vi "Coerce Value.vi"(8 "error in (no error)":errorcluster, 9 "Value":variant, 10 "ParamTags":T1, 11 "Rigol DG822 Pulse in":refnum<class "Rigol DG822 Pulse.lvclass">) -> (0 "error out":errorcluster, 1 "Coerced Value":variant, 3 "Rigol DG822 Pulse out":refnum<class "Rigol DG822 Pulse.lvclass">)   [LabVIEW 2021, in "Rigol DG822 UI.lvlib" / "Rigol DG822 Pulse.lvlib" / "Rigol DG822 Pulse.lvclass"]
uses:
  Rigol DG822 Pulse.lvclass
  Rigol DG822 UI/lib/controls.llb/WaveformParamTags.ctl
  Rigol DG822 UI/lib/controls.llb/FreqUnit.ctl
  Rigol DG822 UI/lib/controls.llb/PeriodUnit.ctl
  Rigol DG822 Pulse.lvclass/Rigol DG822 Pulse.ctl
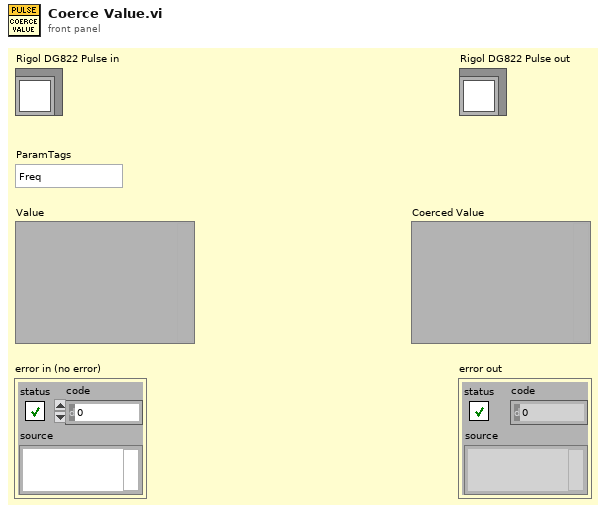
[diagram p1: front panel]
types:
  T1 = typedef "WaveformParamTags.ctl" = enum16{"Freq", "Period", "Ampl", "HighL", "Offset", "LowL", "Phase", "Duty", "Width", "RisEdge", "FallEdge"}
  T2 = typedef "FreqUnit.ctl" = enum32{"No Selection", "MHz", "kHz", "Hz", "mHz", "uHz"}
  T3 = cluster{"Freq":dbl, "FreqUnit":T2, "FreqUnitPrecision":dbl}
  T4 = typedef "PeriodUnit.ctl" = enum32{"No Selection", "s", "ms", "us", "ns"}
  T5 = cluster{"Period":dbl, "PeriodUnit":T4, "PeriodUnitPrecision":dbl}
  T6 = cluster{"Ampl":dbl, "AmplUnit":enum32{"No Selection", "Vpp", "mVpp"}, "AmplUnitPrecision":dbl}
  T7 = cluster{"HighL":dbl, "HighLUnit":enum32{"No Selection", "V", "mV"}, "HighLUnitPrecision":dbl}
  T8 = cluster{"Offset":dbl, "OffsetUnit":enum32{"No Selection", "Vdc", "mVdc"}, "OffsetUnitPrecision":dbl}
  T9 = cluster{"LowL":dbl, "LowLUnit":enum32{"No Selection", "V", "mV"}, "LowLUnitPrecision":dbl}
  T10 = cluster{"Phase":dbl, "PhaseUnit":enum32{"°"}, "PhaseUnitPrecision":dbl}
  T11 = cluster{"Duty":dbl, "DutyUnit":enum32{"%"}, "DutyUnitPrcs":dbl}
  T12 = cluster{"Width":dbl, "WidthUnit":enum32{"No Selection", "s", "ms", "us", "ns"}, "WidthUnitPrcs":dbl}
  T13 = cluster{"RisEdge":dbl, "RisEdgeUnit":enum32{"No Selection", "s", "ms", "us", "ns"}, "RisEdgeUnitPrcs":dbl}
  T14 = cluster{"FallEdge":dbl, "FallEdgeUnit":enum32{"No Selection", "s", "ms", "us", "ns"}, "FallEdgeUnitPrcs":dbl}
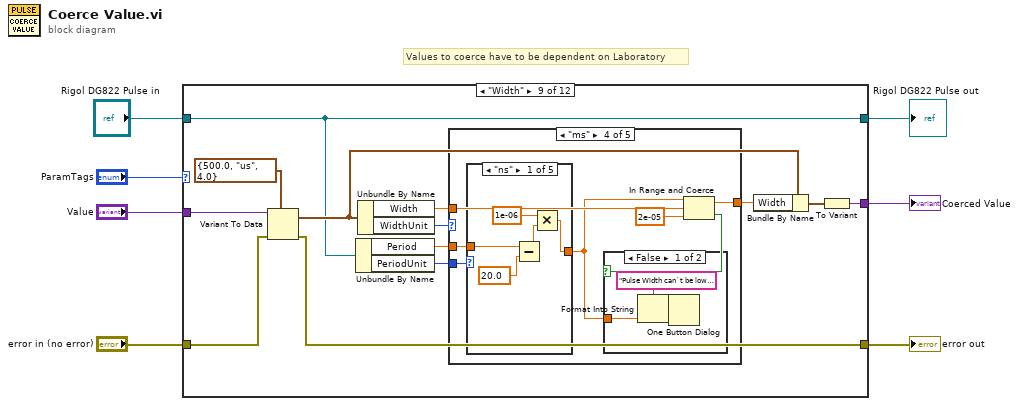
[diagram p0: block diagram]
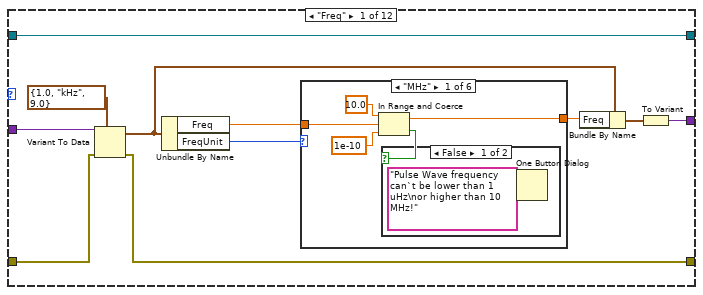
[diagram p2: hidden frame]
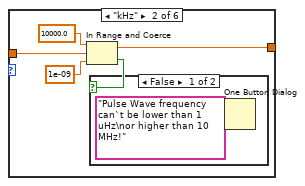
[diagram p4: hidden frame]
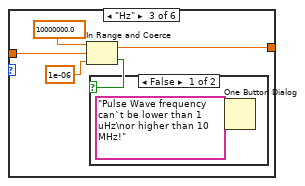
[diagram p6: hidden frame]
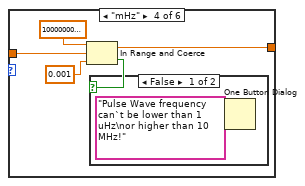
[diagram p8: hidden frame]
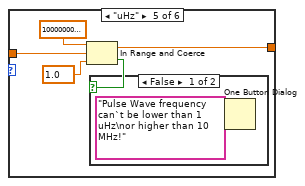
[diagram p10: hidden frame]
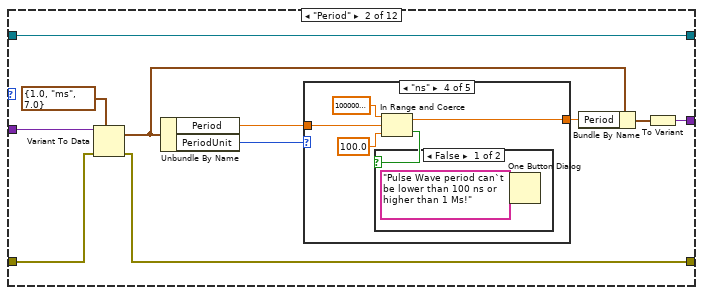
[diagram p13: hidden frame]
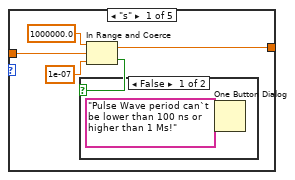
[diagram p14: hidden frame]
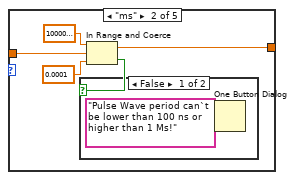
[diagram p16: hidden frame]
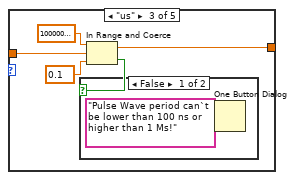
[diagram p18: hidden frame]
diagram:
  # "Values to coerce have to be dependent on Laboratory"
  n1 = case shown="\"Width\"" "ParamTags" {
    tunnel: "Value" -> [w14 w57 w93 w119 w167 w233 w279 w298 w370 w509 w1204 w1886]
    tunnel: "error in (no error)" -> [w12 w53 w90 w117 w165 w231 w276 w296 w368 w507 w1202 w1885]
    tunnel: [w11 w52 w89 w116 w164 w230 w275 w295 w367 w506 w1201 w1885] -> w4
    tunnel: [w9 w50 w87 w114 w162 w228 w273 w293 w365 w504 w1199 w1886] -> w1
    tunnel: "Rigol DG822 Pulse in" -> [w8 w54 w91 w112 w160 w227 w277 w291 w361 w502 w1198 w1887]
    tunnel: [w8 w54 w91 w112 w160 w227 w277 w291 w361 w502 w1198 w1887] -> w2
    frame "Freq" {
      n2 = Variant To Data(error in=w12, type=T3 {"Freq"=1.0, "FreqUnit"=enum."kHz", "FreqUnitPrecision"=9.0} ("Freq"), Variant=w14) -> (data=w13:T3, error out=w11:errorcluster)
      n3 = Unbundle By Name(w13) -> ("Freq"=w17:dbl, "FreqUnit"=w18:T2)
      n4 = case shown="\"MHz\"" w18 {
        tunnel: [w20 w26 w32 w38 w44 w49] -> w16
        tunnel: w17 -> [w21 w27 w33 w39 w45 w49]
        frame "MHz" {
          n5 = In Range and Coerce(upper limit=10.0, x=w21, lower limit=1e-10 ("t")) -> (coerced(x)=w20:dbl, In Range?=w19:bool)
          n6 = case shown="False" w19 {
            frame False {
              n7 = One Button Dialog(message="Pulse Wave frequency can`t be lower than 1 uHz\nor higher than 10 MHz!") -> ()  [unwired: 1 in, 1 out]
            }
            frame True {
            }
          }
        }
        frame "kHz" {
          n8 = In Range and Coerce(upper limit=10000.0, x=w27, lower limit=1e-09 ("t")) -> (coerced(x)=w26:dbl, In Range?=w25:bool)
          n9 = case shown="False" w25 {
            frame False {
              n10 = One Button Dialog(message="Pulse Wave frequency can`t be lower than 1 uHz\nor higher than 10 MHz!") -> ()  [unwired: 1 in, 1 out]
            }
            frame True {
            }
          }
        }
        frame "Hz" {
          n11 = In Range and Coerce(upper limit=10000000.0, x=w33, lower limit=1e-06 ("t")) -> (coerced(x)=w32:dbl, In Range?=w31:bool)
          n12 = case shown="False" w31 {
            frame False {
              n13 = One Button Dialog(message="Pulse Wave frequency can`t be lower than 1 uHz\nor higher than 10 MHz!") -> ()  [unwired: 1 in, 1 out]
            }
            frame True {
            }
          }
        }
        frame "mHz" {
          n14 = In Range and Coerce(upper limit=10000000000.0, x=w39, lower limit=0.001 ("t")) -> (coerced(x)=w38:dbl, In Range?=w37:bool)
          n15 = case shown="False" w37 {
            frame False {
              n16 = One Button Dialog(message="Pulse Wave frequency can`t be lower than 1 uHz\nor higher than 10 MHz!") -> ()  [unwired: 1 in, 1 out]
            }
            frame True {
            }
          }
        }
        frame "uHz" {
          n17 = In Range and Coerce(upper limit=10000000000000.0, x=w45, lower limit=1.0 ("t")) -> (coerced(x)=w44:dbl, In Range?=w43:bool)
          n18 = case shown="False" w43 {
            frame False {
              n19 = One Button Dialog(message="Pulse Wave frequency can`t be lower than 1 uHz\nor higher than 10 MHz!") -> ()  [unwired: 1 in, 1 out]
            }
            frame True {
            }
          }
        }
        frame Default {
        }
      }
      n20 = Bundle By Name(cluster=w13, "Freq"=w16) -> (w10:T3)
      n21 = To Variant(anything=w10) -> (Variant=w9:variant)
    }
    frame "Period" {
      n22 = Variant To Data(error in=w53, type=T5 {"Period"=1.0, "PeriodUnit"=enum."ms", "PeriodUnitPrecision"=7.0} ("Period"), Variant=w57) -> (data=w56:T5, error out=w52:errorcluster)
      n23 = Unbundle By Name(w56) -> ("Period"=w59:dbl, "PeriodUnit"=w60:T4)
      n24 = case shown="\"ns\"" w60 {
        tunnel: [w62 w68 w74 w80 w85] -> w58
        tunnel: w59 -> [w63 w69 w75 w81 w85]
        frame "s" {
          n25 = In Range and Coerce(upper limit=1000000.0, x=w63, lower limit=1e-07 ("t")) -> (coerced(x)=w62:dbl, In Range?=w61:bool)
          n26 = case shown="False" w61 {
            frame False {
              n27 = One Button Dialog(message="Pulse Wave period can`t be lower than 100 ns or higher than 1 Ms!") -> ()  [unwired: 1 in, 1 out]
            }
            frame True {
            }
          }
        }
        frame "ms" {
          n28 = In Range and Coerce(upper limit=1000000000.0, x=w69, lower limit=0.0001 ("t")) -> (coerced(x)=w68:dbl, In Range?=w67:bool)
          n29 = case shown="False" w67 {
            frame False {
              n30 = One Button Dialog(message="Pulse Wave period can`t be lower than 100 ns or higher than 1 Ms!") -> ()  [unwired: 1 in, 1 out]
            }
            frame True {
            }
          }
        }
        frame "us" {
          n31 = In Range and Coerce(upper limit=1000000000000.0, x=w75, lower limit=0.1 ("t")) -> (coerced(x)=w74:dbl, In Range?=w73:bool)
          n32 = case shown="False" w73 {
            frame False {
              n33 = One Button Dialog(message="Pulse Wave period can`t be lower than 100 ns or higher than 1 Ms!") -> ()  [unwired: 1 in, 1 out]
            }
            frame True {
            }
          }
        }
        frame "ns" {
          n34 = In Range and Coerce(upper limit=1000000000000000.0, x=w81, lower limit=100.0 ("t")) -> (coerced(x)=w80:dbl, In Range?=w79:bool)
          n35 = case shown="False" w79 {
            frame False {
              n36 = One Button Dialog(message="Pulse Wave period can`t be lower than 100 ns or higher than 1 Ms!") -> ()  [unwired: 1 in, 1 out]
            }
            frame True {
            }
          }
        }
        frame Default {
        }
      }
      n37 = Bundle By Name(cluster=w56, "Period"=w58) -> (w51:T5)
      n38 = To Variant(anything=w51) -> (Variant=w50:variant)
    }
    frame "Ampl" {
      n39 = Variant To Data(error in=w90, type=T6 {"Ampl"=5.0, "AmplUnit"=enum."Vpp", "AmplUnitPrecision"=4.0} ("Ampl"), Variant=w93) -> (data=w92:T6, error out=w89:errorcluster)
      n40 = Unbundle By Name(w92) -> ("Ampl"=w95:dbl, "AmplUnit"=w96:enum32{"No Selection", "Vpp", "mVpp"})
      n41 = case shown="\"mVpp\"" w96 {
        tunnel: [w99 w105 w109] -> w94
        tunnel: w95 -> [w100 w106 w109]
        frame "Vpp" {
          n42 = In Range and Coerce(upper limit=10.0, x=w100, lower limit=0.002 ("t")) -> (coerced(x)=w99:dbl, In Range?=w97:bool)
          n43 = case shown="False" w97 {
            frame False {
              n44 = One Button Dialog(message="Amplitude can`t be lower than 2 mVpp\nor higher than 10 Vpp!") -> ()  [unwired: 1 in, 1 out]
            }
            frame True {
            }
          }
        }
        frame "mVpp" {
          n45 = In Range and Coerce(upper limit=10000.0, x=w106, lower limit=2.0 ("t")) -> (coerced(x)=w105:dbl, In Range?=w103:bool)
          n46 = case shown="False" w103 {
            frame False {
              n47 = One Button Dialog(message="Amplitude can`t be lower than 2 mVpp\nor higher than 10 Vpp!") -> ()  [unwired: 1 in, 1 out]
            }
            frame True {
            }
          }
        }
        frame Default {
        }
      }
      n48 = Bundle By Name(cluster=w92, "Ampl"=w94) -> (w88:T6)
      n49 = To Variant(anything=w88) -> (Variant=w87:variant)
    }
    frame "HighL" {
      n50 = Variant To Data(error in=w117, type=T7 {"HighL"=2.5, "HighLUnit"=enum."V", "HighLUnitPrecision"=4.0} ("HighL"), Variant=w119) -> (data=w118:T7, error out=w116:errorcluster)
      n51 = Unbundle By Name(w118) -> ("HighL"=w121:dbl, "HighLUnit"=w122:enum32{"No Selection", "V", "mV"})
      n52 = Unbundle By Name(w112) -> ("LowL"=w111:dbl, "LowLUnit"=w110:enum32{"No Selection", "V", "mV"})
      n53 = case shown="\"V\"" w122 {
        tunnel: [w127 w144 w157] -> w120
        tunnel: w121 -> [w128 w145 w157]
        tunnel: w111 -> [w123 w140 _]
        tunnel: w110 -> [w125 w142 _]
        frame "V" {
          n54 = case shown="\"V\"" w125 {
            tunnel: [w130 w136 w138] -> w124
            tunnel: w123 -> [w132 w137 w138]
            frame "V" {
              n55 = Add(x=w132, y=0.002 ("upper limit")) -> (x+y=w130:dbl)
            }
            frame "mV" {
              n56 = Divide(x=w137, y=1000.0) -> (x/y=w135:dbl)
              n57 = Add(x=w135, y=0.002 ("upper limit")) -> (x+y=w136:dbl)
            }
            frame Default {
            }
          }
          n58 = In Range and Coerce(upper limit=5.0, x=w128, lower limit=w124) -> (coerced(x)=w127:dbl, In Range?=w126:bool)
          n59 = case shown="False" w126 {
            frame False {
              n60 = One Button Dialog(message="HighL can`t be higher than 5 V or less than 2 mV higher than LowL!\n") -> ()  [unwired: 1 in, 1 out]
            }
            frame True {
            }
          }
        }
        frame "mV" {
          n61 = case shown="\"mV\"" w142 {
            tunnel: [w150 w154 w155] -> w141
            tunnel: w140 -> [w149 w152 w155]
            frame "V" {
              n62 = Multiply(x=w149, y=1000.0) -> (x*y=w147:dbl)
              n63 = Add(x=w147, y=2.0 ("upper limit")) -> (x+y=w150:dbl)
            }
            frame "mV" {
              n64 = Add(x=w152, y=2.0 ("upper limit")) -> (x+y=w154:dbl)
            }
            frame Default {
            }
          }
          n65 = In Range and Coerce(upper limit=5000.0, x=w145, lower limit=w141) -> (coerced(x)=w144:dbl, In Range?=w143:bool)
          n66 = case shown="False" w143 {
            frame False {
              n67 = One Button Dialog(message="HighL can`t be higher than 5 V or less than 2 mV higher than LowL!\n") -> ()  [unwired: 1 in, 1 out]
            }
            frame True {
            }
          }
        }
        frame Default {
        }
      }
      n68 = Bundle By Name(cluster=w118, "HighL"=w120) -> (w115:T7)
      n69 = To Variant(anything=w115) -> (Variant=w114:variant)
    }
    frame "Offset" {
      n70 = Variant To Data(error in=w165, type=T8 {"Offset"=0.0, "OffsetUnit"=enum."Vdc", "OffsetUnitPrecision"=4.0} ("Offset"), Variant=w167) -> (data=w166:T8, error out=w164:errorcluster)
      n71 = Unbundle By Name(w166) -> ("Offset"=w169:dbl, "OffsetUnit"=w170:enum32{"No Selection", "Vdc", "mVdc"})
      n72 = Unbundle By Name(w160) -> ("Ampl"=w159:dbl, "AmplUnit"=w158:enum32{"No Selection", "Vpp", "mVpp"})
      n73 = case shown="\"mVdc\"" w170 {
        tunnel: [w176 w202 w223] -> w168
        tunnel: w169 -> [w177 w203 w223]
        tunnel: w159 -> [w173 w199 _]
        tunnel: w158 -> [w174 w200 _]
        frame "Vdc" {
          n74 = case shown="\"Vpp\"" w174 {
            tunnel: w173 -> [w184 w192 _]
            tunnel: [w179 w187 5.0] -> w172
            tunnel: [w178 w186 -5.0] -> w171
            frame "Vpp" {
              w180 = 2.0 ("t")
              n75 = Add(x=w184, y=-10.0 ("t")) -> (x+y=w182:dbl)
              n76 = Subtract(x=10.0 ("t"), y=w184) -> (x-y=w181:dbl)
              n77 = Divide(x=w182, y=w180) -> (x/y=w178:dbl)
              n78 = Divide(x=w181, y=w180) -> (x/y=w179:dbl)
            }
            frame "mVpp" {
              w188 = 2000.0 ("t")
              n79 = Add(x=w192, y=-10000.0 ("t")) -> (x+y=w190:dbl)
              n80 = Subtract(x=10000.0 ("t"), y=w192) -> (x-y=w189:dbl)
              n81 = Divide(x=w190, y=w188) -> (x/y=w186:dbl)
              n82 = Divide(x=w189, y=w188) -> (x/y=w187:dbl)
            }
            frame Default {
            }
          }
          n83 = In Range and Coerce(upper limit=w172, x=w177, lower limit=w171) -> (coerced(x)=w176:dbl, In Range?=w175:bool)
          n84 = case shown="False" w175 {
            frame False {
              n85 = One Button Dialog(message="Offset upper and lower limit can`t exceed (10 - Ampl)/2 value") -> ()  [unwired: 1 in, 1 out]
            }
            frame True {
            }
          }
        }
        frame "mVdc" {
          n86 = case shown="\"Vpp\"" w200 {
            tunnel: w199 -> [w210 w218 _]
            tunnel: [w205 w213 5.0] -> w198
            tunnel: [w204 w212 -5.0] -> w197
            frame "Vpp" {
              w206 = 0.002 ("t")
              n87 = Add(x=w210, y=-10.0 ("t")) -> (x+y=w208:dbl)
              n88 = Subtract(x=10.0 ("t"), y=w210) -> (x-y=w207:dbl)
              n89 = Divide(x=w208, y=w206) -> (x/y=w204:dbl)
              n90 = Divide(x=w207, y=w206) -> (x/y=w205:dbl)
            }
            frame "mVpp" {
              w214 = 2.0 ("t")
              n91 = Add(x=w218, y=-10000.0 ("t")) -> (x+y=w216:dbl)
              n92 = Subtract(x=10000.0 ("t"), y=w218) -> (x-y=w215:dbl)
              n93 = Divide(x=w216, y=w214) -> (x/y=w212:dbl)
              n94 = Divide(x=w215, y=w214) -> (x/y=w213:dbl)
            }
            frame Default {
            }
          }
          n95 = In Range and Coerce(upper limit=w198, x=w203, lower limit=w197) -> (coerced(x)=w202:dbl, In Range?=w201:bool)
          n96 = case shown="False" w201 {
            frame False {
              n97 = One Button Dialog(message="Offset upper and lower limit can`t exceed (10 - Ampl)/2 value") -> ()  [unwired: 1 in, 1 out]
            }
            frame True {
            }
          }
        }
        frame Default {
        }
      }
      n98 = Bundle By Name(cluster=w166, "Offset"=w168) -> (w163:T8)
      n99 = To Variant(anything=w163) -> (Variant=w162:variant)
    }
    frame "LowL" {
      n100 = Variant To Data(error in=w231, type=T9 {"LowL"=-2.5, "LowLUnit"=enum."V", "LowLUnitPrecision"=4.0} ("LowL"), Variant=w233) -> (data=w232:T9, error out=w230:errorcluster)
      n101 = Unbundle By Name(w232) -> ("LowL"=w235:dbl, "LowLUnit"=w236:enum32{"No Selection", "V", "mV"})
      n102 = Unbundle By Name(w227) -> ("HighL"=w226:dbl, "HighLUnit"=w225:enum32{"No Selection", "V", "mV"})
      n103 = case shown="\"mV\"" w236 {
        tunnel: [w242 w259 w271] -> w234
        tunnel: w235 -> [w243 w260 w271]
        tunnel: w226 -> [w239 w256 _]
        tunnel: w225 -> [w240 w257 _]
        frame "V" {
          n104 = case shown="\"mV\"" w240 {
            tunnel: [w244 w250 w252] -> w237
            tunnel: w239 -> [w246 w251 w252]
            frame "V" {
              n105 = Subtract(x=w246, y=0.002 ("upper limit")) -> (x-y=w244:dbl)
            }
            frame "mV" {
              n106 = Divide(x=w251, y=1000.0) -> (x/y=w249:dbl)
              n107 = Subtract(x=w249, y=0.002 ("upper limit")) -> (x-y=w250:dbl)
            }
            frame Default {
            }
          }
          n108 = In Range and Coerce(upper limit=w237, x=w243, lower limit=-5.0 ("upper limit")) -> (coerced(x)=w242:dbl, In Range?=w241:bool)
          n109 = case shown="False" w241 {
            frame False {
              n110 = One Button Dialog(message="LowL can`t be lower  than -5 V or less than 2 mV lower than HighL!") -> ()  [unwired: 1 in, 1 out]
            }
            frame True {
            }
          }
        }
        frame "mV" {
          n111 = case shown="\"V\"" w257 {
            tunnel: [w264 w268 w269] -> w254
            tunnel: w256 -> [w263 w266 w269]
            frame "V" {
              n112 = Multiply(x=w263, y=1000.0) -> (x*y=w261:dbl)
              n113 = Subtract(x=w261, y=2.0 ("upper limit")) -> (x-y=w264:dbl)
            }
            frame "mV" {
              n114 = Subtract(x=w266, y=2.0 ("upper limit")) -> (x-y=w268:dbl)
            }
            frame Default {
            }
          }
          n115 = In Range and Coerce(upper limit=w254, x=w260, lower limit=-5000.0 ("upper limit")) -> (coerced(x)=w259:dbl, In Range?=w258:bool)
          n116 = case shown="False" w258 {
            frame False {
              n117 = One Button Dialog(message="LowL can`t be lower  than -5 V or less than 2 mV lower than HighL!") -> ()  [unwired: 1 in, 1 out]
            }
            frame True {
            }
          }
        }
        frame Default {
        }
      }
      n118 = Bundle By Name(cluster=w232, "LowL"=w234) -> (w229:T9)
      n119 = To Variant(anything=w229) -> (Variant=w228:variant)
    }
    frame "Phase" {
      n120 = Variant To Data(error in=w276, type=T10 {"Phase"=0.0, "PhaseUnit"=enum."°", "PhaseUnitPrecision"=3.0} ("Phase"), Variant=w279) -> (data=w278:T10, error out=w275:errorcluster)
      n121 = Unbundle By Name(w278) -> ("Phase"=w281:dbl, "PhaseUnit"=w282:enum32{"°"})
      n122 = case shown="\"°\"" w282 {
        tunnel: [w283 w284] -> w280
        tunnel: w281 -> [w283 w285]
        frame Default {
        }
        frame "°" {
          n123 = Quotient & Remainder(x=w285, y=360.0) -> (x-y*floor(x/y)=w284:dbl)  [unwired: 1 out]
        }
      }
      n124 = Bundle By Name(cluster=w278, "Phase"=w280) -> (w274:T10)
      n125 = To Variant(anything=w274) -> (Variant=w273:variant)
    }
    frame "Duty" {
      n126 = Variant To Data(error in=w296, type=T11 {"Duty"=50.0, "DutyUnit"=enum."%", "DutyUnitPrcs"=3.0} ("Duty"), Variant=w298) -> (data=w297:T11, error out=w295:errorcluster)
      n127 = Unbundle By Name(w291) -> ("PeriodUnit"=w287:enum32{"No Selection", "s", "ms", "us", "ns"}, "Period"=w288:dbl)
      n128 = Unbundle By Name(w297) -> ("Duty"=w289:dbl)
      n129 = case shown="\"s\"" w287 {
        tunnel: [w299 w308 w325 w342 w354] -> w290
        tunnel: w289 -> [w299 w307 w324 w341 w353]
        tunnel: w288 -> [_ w302 w319 w336 _]
        frame Default {
        }
        frame "ns" {
          w301 = 2000.0 ("lower limit")
          n130 = Multiply(x=100.0 ("y"), y=w302) -> (x*y=w309:dbl)
          n131 = Multiply(x=w307, y=w302) -> (x*y=w311:dbl)
          n132 = Divide(x=w301, y=w302) -> (x/y=w303:dbl)
          n133 = Subtract(x=w309, y=w301) -> (x-y=w300:dbl)
          n134 = Divide(x=w300, y=w302) -> (x/y=w304:dbl)
          n135 = In Range and Coerce(upper limit=w300, x=w311, lower limit=w301) -> (coerced(x)=w310:dbl, In Range?=w305:bool)
          n136 = case shown="False" w305 {
            tunnel: w303 -> [w315 _]
            tunnel: w304 -> [w312 _]
            frame False {
              w313 = "%" ("input 2")
              n137 = Format Into String(format string="Duty Cycle can`t be lower than %.3f %s\nor higher than %.3f %s!" ("message"), w315, w313, w312, w313) -> (resulting string=w316:string)  [unwired: 2 in, 1 out]
              n138 = One Button Dialog(message=w316) -> ()  [unwired: 1 in, 1 out]
            }
            frame True {
            }
          }
          n139 = Divide(x=w310, y=w302) -> (x/y=w308:dbl)
        }
        frame "us" {
          w318 = 2.0 ("lower limit")
          n140 = Multiply(x=100.0 ("y"), y=w319) -> (x*y=w326:dbl)
          n141 = Multiply(x=w324, y=w319) -> (x*y=w328:dbl)
          n142 = Divide(x=w318, y=w319) -> (x/y=w320:dbl)
          n143 = Subtract(x=w326, y=w318) -> (x-y=w317:dbl)
          n144 = Divide(x=w317, y=w319) -> (x/y=w321:dbl)
          n145 = In Range and Coerce(upper limit=w317, x=w328, lower limit=w318) -> (coerced(x)=w327:dbl, In Range?=w322:bool)
          n146 = case shown="False" w322 {
            tunnel: w320 -> [w332 _]
            tunnel: w321 -> [w329 _]
            frame False {
              w330 = "%" ("input 2")
              n147 = Format Into String(format string="Duty Cycle can`t be lower than %.3f %s\nor higher than %.3f %s!" ("message"), w332, w330, w329, w330) -> (resulting string=w333:string)  [unwired: 2 in, 1 out]
              n148 = One Button Dialog(message=w333) -> ()  [unwired: 1 in, 1 out]
            }
            frame True {
            }
          }
          n149 = Divide(x=w327, y=w319) -> (x/y=w325:dbl)
        }
        frame "ms" {
          w335 = 0.002 ("lower limit")
          n150 = Multiply(x=100.0 ("y"), y=w336) -> (x*y=w343:dbl)
          n151 = Multiply(x=w341, y=w336) -> (x*y=w345:dbl)
          n152 = Divide(x=w335, y=w336) -> (x/y=w337:dbl)
          n153 = Subtract(x=w343, y=w335) -> (x-y=w334:dbl)
          n154 = Divide(x=w334, y=w336) -> (x/y=w338:dbl)
          n155 = In Range and Coerce(upper limit=w334, x=w345, lower limit=w335) -> (coerced(x)=w344:dbl, In Range?=w339:bool)
          n156 = case shown="False" w339 {
            tunnel: w337 -> [w349 _]
            tunnel: w338 -> [w346 _]
            frame False {
              w347 = "%" ("input 2")
              n157 = Format Into String(format string="Duty Cycle can`t be lower than %.3f %s\nor higher than %.3f %s!" ("message"), w349, w347, w346, w347) -> (resulting string=w350:string)  [unwired: 2 in, 1 out]
              n158 = One Button Dialog(message=w350) -> ()  [unwired: 1 in, 1 out]
            }
            frame True {
            }
          }
          n159 = Divide(x=w344, y=w336) -> (x/y=w342:dbl)
        }
        frame "s" {
          w352 = 0.005 ("lower limit")
          w351 = 99.995 ("upper limit")
          n160 = In Range and Coerce(upper limit=w351, x=w353, lower limit=w352) -> (coerced(x)=w354:dbl, In Range?=w355:bool)
          n161 = case shown="False" w355 {
            tunnel: w352 -> [w359 _]
            tunnel: w351 -> [w356 _]
            frame False {
              w357 = "%" ("input 2")
              n162 = Format Into String(format string="Duty Cycle can`t be lower than %.3f %s\nor higher than %.3f %s!" ("message"), w359, w357, w356, w357) -> (resulting string=w360:string)  [unwired: 2 in, 1 out]
              n163 = One Button Dialog(message=w360) -> ()  [unwired: 1 in, 1 out]
            }
            frame True {
            }
          }
        }
      }
      n164 = Bundle By Name(cluster=w297, "Duty"=w290) -> (w294:T11)
      n165 = To Variant(anything=w294) -> (Variant=w293:variant)
    }
    frame "Width" {
      n166 = Variant To Data(error in=w368, type=T12 {"Width"=500.0, "WidthUnit"=enum."us", "WidthUnitPrcs"=4.0} ("Width"), Variant=w370) -> (data=w369:T12, error out=w367:errorcluster)
      n167 = Unbundle By Name(w361) -> ("Period"=w364:dbl, "PeriodUnit"=w363:enum32{"No Selection", "s", "ms", "us", "ns"})
      n168 = Unbundle By Name(w369) -> ("Width"=w372:dbl, "WidthUnit"=w373:enum32{"No Selection", "s", "ms", "us", "ns"})
      n169 = case shown="\"ms\"" w373 {
        tunnel: [w374 w380 w411 w442 w476] -> w371
        tunnel: w372 -> [w374 w381 w412 w443 w477]
        tunnel: w364 -> [_ w378 w409 w440 w474]
        tunnel: w363 -> [_ w379 w410 w441 w475]
        frame Default {
        }
        frame "ns" {
          w376 = 20.0 ("lower limit")
          n170 = case shown="\"s\"" w379 {
            tunnel: w378 -> [w388 w393 w398 w403 _]
            tunnel: [w387 w392 w397 w402 -1.0] -> w375
            frame "ns" {
              n171 = Subtract(x=w388, y=20.0 ("x")) -> (x-y=w387:dbl)
            }
            frame "us" {
              n172 = Subtract(x=w393, y=0.02 ("x")) -> (x-y=w391:dbl)
              n173 = Multiply(x=1000.0, y=w391) -> (x*y=w392:dbl)
            }
            frame "ms" {
              n174 = Subtract(x=w398, y=2e-05 ("x")) -> (x-y=w396:dbl)
              n175 = Multiply(x=1000000.0, y=w396) -> (x*y=w397:dbl)
            }
            frame "s" {
              n176 = Subtract(x=w403, y=2e-08 ("x")) -> (x-y=w401:dbl)
              n177 = Multiply(x=1000000000.0, y=w401) -> (x*y=w402:dbl)
            }
            frame Default {
            }
          }
          n178 = In Range and Coerce(upper limit=w375, x=w381, lower limit=w376) -> (coerced(x)=w380:dbl, In Range?=w377:bool)
          n179 = case shown="False" w377 {
            tunnel: w376 -> [w385 _]
            tunnel: w375 -> [w382 _]
            frame False {
              w383 = "ns" ("input 2")
              n180 = Format Into String(format string="Pulse Width can`t be lower than %.3f %s or higher than %.3f %s!" ("message"), w385, w383, w382, w383) -> (resulting string=w386:string)  [unwired: 2 in, 1 out]
              n181 = One Button Dialog(message=w386) -> ()  [unwired: 1 in, 1 out]
            }
            frame True {
            }
          }
        }
        frame "us" {
          n182 = case shown="\"s\"" w410 {
            tunnel: w409 -> [w419 w424 w429 w434 _]
            tunnel: [w417 w423 w428 w433 -1.0] -> w406
            frame "ns" {
              n183 = Subtract(x=w419, y=20.0 ("x")) -> (x-y=w416:dbl)
              n184 = Multiply(x=0.001, y=w416) -> (x*y=w417:dbl)
            }
            frame "us" {
              n185 = Subtract(x=w424, y=0.02 ("x")) -> (x-y=w422:dbl)
              n186 = Multiply(x=1.0, y=w422) -> (x*y=w423:dbl)
            }
            frame "ms" {
              n187 = Subtract(x=w429, y=2e-05 ("x")) -> (x-y=w427:dbl)
              n188 = Multiply(x=1000.0, y=w427) -> (x*y=w428:dbl)
            }
            frame "s" {
              n189 = Subtract(x=w434, y=2e-08 ("x")) -> (x-y=w432:dbl)
              n190 = Multiply(x=1000000.0, y=w432) -> (x*y=w433:dbl)
            }
            frame Default {
            }
          }
          n191 = In Range and Coerce(upper limit=w406, x=w412, lower limit=0.02) -> (coerced(x)=w411:dbl, In Range?=w408:bool)
          n192 = case shown="False" w408 {
            tunnel: w406 -> [w413 _]
            frame False {
              n193 = Format Into String(format string="Pulse Width can`t be lower than 20 ns or higher than %.3f us!" ("message"), w413) -> (resulting string=w415:string)  [unwired: 2 in, 1 out]
              n194 = One Button Dialog(message=w415) -> ()  [unwired: 1 in, 1 out]
            }
            frame True {
            }
          }
        }
        frame "ms" {
          n195 = case shown="\"ns\"" w441 {
            tunnel: w440 -> [w450 w455 w460 w465 _]
            tunnel: [w448 w454 w459 w464 -1.0] -> w437
            frame "ns" {
              n196 = Subtract(x=w450, y=20.0 ("x")) -> (x-y=w447:dbl)
              n197 = Multiply(x=1e-06, y=w447) -> (x*y=w448:dbl)
            }
            frame "us" {
              n198 = Subtract(x=w455, y=0.02 ("x")) -> (x-y=w453:dbl)
              n199 = Multiply(x=0.001, y=w453) -> (x*y=w454:dbl)
            }
            frame "ms" {
              n200 = Subtract(x=w460, y=2e-05 ("x")) -> (x-y=w458:dbl)
              n201 = Multiply(x=1.0, y=w458) -> (x*y=w459:dbl)
            }
            frame "s" {
              n202 = Subtract(x=w465, y=2e-08 ("x")) -> (x-y=w463:dbl)
              n203 = Multiply(x=1000.0, y=w463) -> (x*y=w464:dbl)
            }
            frame Default {
            }
          }
          n204 = In Range and Coerce(upper limit=w437, x=w443, lower limit=2e-05) -> (coerced(x)=w442:dbl, In Range?=w439:bool)
          n205 = case shown="False" w439 {
            tunnel: w437 -> [w444 _]
            frame False {
              n206 = Format Into String(format string="Pulse Width can`t be lower than 20 ns or higher than %.3f ms!" ("message"), w444) -> (resulting string=w446:string)  [unwired: 2 in, 1 out]
              n207 = One Button Dialog(message=w446) -> ()  [unwired: 1 in, 1 out]
            }
            frame True {
            }
          }
        }
        frame "s" {
          n208 = case shown="\"s\"" w475 {
            tunnel: w474 -> [w482 w485 w488 w491 _]
            tunnel: [w483 w487 w490 w493 -1.0] -> w472
            frame "ns" {
              n209 = Multiply(x=1e-09, y=w482) -> (x*y=w483:dbl)
            }
            frame "us" {
              n210 = Multiply(x=1e-06, y=w485) -> (x*y=w487:dbl)
            }
            frame "ms" {
              n211 = Multiply(x=0.001, y=w488) -> (x*y=w490:dbl)
            }
            frame "s" {
              n212 = Multiply(x=1.0, y=w491) -> (x*y=w493:dbl)
            }
            frame Default {
            }
          }
          n213 = Multiply(x=0.99995 ("upper limit"), y=w472) -> (x*y=w470:dbl)
          n214 = Multiply(x=w472, y=5e-05 ("lower limit")) -> (x*y=w471:dbl)
          n215 = In Range and Coerce(upper limit=w470, x=w477, lower limit=w471) -> (coerced(x)=w476:dbl, In Range?=w473:bool)
          n216 = case shown="False" w473 {
            tunnel: w471 -> [w478 _]
            tunnel: w470 -> [w479 _]
            frame False {
              n217 = Format Into String(format string="Pulse Width can`t be lower than %.3f s or higher than %.3f s!" ("message"), w478, w479) -> (resulting string=w481:string)  [unwired: 2 in, 1 out]
              n218 = One Button Dialog(message=w481) -> ()  [unwired: 1 in, 1 out]
            }
            frame True {
            }
          }
        }
      }
      n219 = Bundle By Name(cluster=w369, "Width"=w371) -> (w366:T12)
      n220 = To Variant(anything=w366) -> (Variant=w365:variant)
    }
    frame "RisEdge" {
      n221 = Variant To Data(error in=w507, type=T13 {"RisEdge"=10.0, "RisEdgeUnit"=enum."ns", "RisEdgeUnitPrcs"=1.0} ("RisEdge"), Variant=w509) -> (data=w508:T13, error out=w506:errorcluster)
      n222 = Unbundle By Name(w508) -> ("RisEdge"=w501:dbl, "RisEdgeUnit"=w500:enum32{"No Selection", "s", "ms", "us", "ns"})
      n223 = Unbundle By Name(w502) -> ("Period"=w497:dbl, "PeriodUnit"=w498:enum32{"No Selection", "s", "ms", "us", "ns"}, "Width"=w496:dbl, "WidthUnit"=w495:enum32{"No Selection", "s", "ms", "us", "ns"})
      n224 = case shown="\"ns\"" w500 {
        tunnel: w501 -> [w510 w520 w688 w858 w1028]
        tunnel: [w510 w521 w689 w859 w1029] -> w499
        tunnel: w498 -> [_ w518 w686 w856 w1026]
        tunnel: w497 -> [_ w517 w685 w855 w1025]
        tunnel: w496 -> [_ w516 w684 w854 w1024]
        tunnel: w495 -> [_ w515 w683 w853 w1023]
        frame Default {
        }
        frame "ns" {
          n225 = case shown="\"s\"" w518 {
            tunnel: w517 -> [_ w536 w573 w612 w651]
            tunnel: w516 -> [w526 w540 w577 w616 w655]
            tunnel: w515 -> [_ w541 w578 w617 w656]
            tunnel: [w526 w528 w566 w605 w644] -> w512
            tunnel: ["ns" "ns" "us" "ms" "s"] -> w514
            tunnel: [w526 w528 w563 w602 w641] -> w511
            frame Default {
            }
            frame "ns" {
              w537 = 0.795 ("lower limit")
              n226 = case shown="\"ns\"" w541 {
                tunnel: w540 -> [w543 w545 w549 w554 w559]
                tunnel: [w544 w546 w551 w556 w561] -> w535
                tunnel: [w543 w545 w548 w553 w558] -> w530
                frame Default {
                  n227 = Multiply(x=w543, y=3.0) -> (x*y=w544:dbl)
                }
                frame "ns" {
                  n228 = Multiply(x=w545, y=3.0) -> (x*y=w546:dbl)
                }
                frame "us" {
                  n229 = Multiply(x=w549, y=1000.0) -> (x*y=w548:dbl)
                  n230 = Multiply(x=w548, y=3.0) -> (x*y=w551:dbl)
                }
                frame "ms" {
                  n231 = Multiply(x=w554, y=1000000.0) -> (x*y=w553:dbl)
                  n232 = Multiply(x=w553, y=3.0) -> (x*y=w556:dbl)
                }
                frame "s" {
                  n233 = Multiply(x=w559, y=1000000000.0) -> (x*y=w558:dbl)
                  n234 = Multiply(x=w558, y=3.0) -> (x*y=w561:dbl)
                }
              }
              n235 = Subtract(x=w536, y=w530) -> (x-y=w534:dbl)
              n236 = Divide(x=w534, y=2.0) -> (x/y=w533:dbl)
              n237 = Multiply(x=w537, y=w533) -> (x*y=w531:dbl)
              n238 = Multiply(x=w537, y=w535) -> (x*y=w538:dbl)
              n239 = Less?(x=w536, y=w535) -> (x < y?=w539:bool)
              n240 = Select(t=w531, s=w539, f=w538) -> (s? t:f=w528:dbl)
            }
            frame "us" {
              w574 = 0.795 ("lower limit")
              n241 = case shown="Default" w578 {
                tunnel: w577 -> [w579 w583 w588 w593 w598]
                tunnel: [w580 w585 w590 w595 w600] -> w572
                tunnel: [w579 w582 w587 w592 w597] -> w567
                frame Default {
                  n242 = Multiply(x=w579, y=3.0) -> (x*y=w580:dbl)
                }
                frame "ns" {
                  n243 = Multiply(x=w583, y=0.001) -> (x*y=w582:dbl)
                  n244 = Multiply(x=w582, y=3.0) -> (x*y=w585:dbl)
                }
                frame "us" {
                  n245 = Multiply(x=w588, y=1.0) -> (x*y=w587:dbl)
                  n246 = Multiply(x=w587, y=3.0) -> (x*y=w590:dbl)
                }
                frame "ms" {
                  n247 = Multiply(x=w593, y=1000.0) -> (x*y=w592:dbl)
                  n248 = Multiply(x=w592, y=3.0) -> (x*y=w595:dbl)
                }
                frame "s" {
                  n249 = Multiply(x=w598, y=1000000.0) -> (x*y=w597:dbl)
                  n250 = Multiply(x=w597, y=3.0) -> (x*y=w600:dbl)
                }
              }
              n251 = Subtract(x=w573, y=w567) -> (x-y=w571:dbl)
              n252 = Divide(x=w571, y=2.0) -> (x/y=w570:dbl)
              n253 = Multiply(x=w574, y=w570) -> (x*y=w568:dbl)
              n254 = Multiply(x=w574, y=w572) -> (x*y=w575:dbl)
              n255 = Less?(x=w573, y=w572) -> (x < y?=w576:bool)
              n256 = Select(t=w568, s=w576, f=w575) -> (s? t:f=w563:dbl)
              n257 = Multiply(x=1000.0, y=w563) -> (x*y=w566:dbl)
            }
            frame "ms" {
              w613 = 0.795 ("lower limit")
              n258 = case shown="\"us\"" w617 {
                tunnel: w616 -> [w618 w622 w627 w632 w637]
                tunnel: [w619 w624 w629 w634 w639] -> w611
                tunnel: [w618 w621 w626 w631 w636] -> w606
                frame Default {
                  n259 = Multiply(x=w618, y=3.0) -> (x*y=w619:dbl)
                }
                frame "ns" {
                  n260 = Multiply(x=w622, y=1e-06) -> (x*y=w621:dbl)
                  n261 = Multiply(x=w621, y=3.0) -> (x*y=w624:dbl)
                }
                frame "us" {
                  n262 = Multiply(x=w627, y=0.001) -> (x*y=w626:dbl)
                  n263 = Multiply(x=w626, y=3.0) -> (x*y=w629:dbl)
                }
                frame "ms" {
                  n264 = Multiply(x=w632, y=1.0) -> (x*y=w631:dbl)
                  n265 = Multiply(x=w631, y=3.0) -> (x*y=w634:dbl)
                }
                frame "s" {
                  n266 = Multiply(x=w637, y=1000.0) -> (x*y=w636:dbl)
                  n267 = Multiply(x=w636, y=3.0) -> (x*y=w639:dbl)
                }
              }
              n268 = Subtract(x=w612, y=w606) -> (x-y=w610:dbl)
              n269 = Divide(x=w610, y=2.0) -> (x/y=w609:dbl)
              n270 = Multiply(x=w613, y=w609) -> (x*y=w607:dbl)
              n271 = Multiply(x=w613, y=w611) -> (x*y=w614:dbl)
              n272 = Less?(x=w612, y=w611) -> (x < y?=w615:bool)
              n273 = Select(t=w607, s=w615, f=w614) -> (s? t:f=w602:dbl)
              n274 = Multiply(x=1000000.0, y=w602) -> (x*y=w605:dbl)
            }
            frame "s" {
              w652 = 0.795 ("lower limit")
              n275 = case shown="Default" w656 {
                tunnel: w655 -> [w658 w661 w666 w671 w676]
                tunnel: [w657 w663 w668 w673 w678] -> w650
                tunnel: [w658 w660 w665 w670 w675] -> w645
                frame Default {
                  n276 = Multiply(x=w658, y=3.0) -> (x*y=w657:dbl)
                }
                frame "ns" {
                  n277 = Multiply(x=w661, y=1e-06) -> (x*y=w660:dbl)
                  n278 = Multiply(x=w660, y=3.0) -> (x*y=w663:dbl)
                }
                frame "us" {
                  n279 = Multiply(x=w666, y=0.001) -> (x*y=w665:dbl)
                  n280 = Multiply(x=w665, y=3.0) -> (x*y=w668:dbl)
                }
                frame "ms" {
                  n281 = Multiply(x=w671, y=1.0) -> (x*y=w670:dbl)
                  n282 = Multiply(x=w670, y=3.0) -> (x*y=w673:dbl)
                }
                frame "s" {
                  n283 = Multiply(x=w676, y=1000.0) -> (x*y=w675:dbl)
                  n284 = Multiply(x=w675, y=3.0) -> (x*y=w678:dbl)
                }
              }
              n285 = Subtract(x=w651, y=w645) -> (x-y=w649:dbl)
              n286 = Divide(x=w649, y=2.0) -> (x/y=w648:dbl)
              n287 = Multiply(x=w652, y=w648) -> (x*y=w646:dbl)
              n288 = Multiply(x=w652, y=w650) -> (x*y=w653:dbl)
              n289 = Less?(x=w651, y=w650) -> (x < y?=w654:bool)
              n290 = Select(t=w646, s=w654, f=w653) -> (s? t:f=w641:dbl)
              n291 = Multiply(x=1000000000.0, y=w641) -> (x*y=w644:dbl)
            }
          }
          n292 = In Range and Coerce(upper limit=w512, x=w520, lower limit=10.0) -> (coerced(x)=w521:dbl, In Range?=w513:bool)
          n293 = case shown="False" w513 {
            tunnel: w511 -> [w523 _]
            tunnel: w514 -> [w522 _]
            frame False {
              n294 = Format Into String(format string="RisEdge time can`t be lower than 10 ns or higher than %.3f %s!" ("message"), w523, w522) -> (resulting string=w525:string)  [unwired: 2 in, 1 out]
              n295 = One Button Dialog(message=w525) -> ()  [unwired: 1 in, 1 out]
            }
            frame True {
            }
          }
        }
        frame "us" {
          n296 = case shown="\"ns\"" w686 {
            tunnel: w685 -> [_ w706 w743 w782 w821]
            tunnel: w684 -> [w695 w710 w747 w786 w825]
            tunnel: w683 -> [_ w711 w748 w787 w826]
            tunnel: [w695 w698 w736 w775 w814] -> w681
            tunnel: ["ns" "ns" "us" "ms" "s"] -> w680
            frame Default {
            }
            frame "ns" {
              w707 = 0.795 ("lower limit")
              n297 = case shown="Default" w711 {
                tunnel: w710 -> [w712 w715 w719 w724 w729]
                tunnel: [w713 w716 w721 w726 w731] -> w705
                tunnel: [w712 w715 w718 w723 w728] -> w700
                frame Default {
                  n298 = Multiply(x=w712, y=3.0) -> (x*y=w713:dbl)
                }
                frame "ns" {
                  n299 = Multiply(x=w715, y=3.0) -> (x*y=w716:dbl)
                }
                frame "us" {
                  n300 = Multiply(x=w719, y=1000.0) -> (x*y=w718:dbl)
                  n301 = Multiply(x=w718, y=3.0) -> (x*y=w721:dbl)
                }
                frame "ms" {
                  n302 = Multiply(x=w724, y=1000000.0) -> (x*y=w723:dbl)
                  n303 = Multiply(x=w723, y=3.0) -> (x*y=w726:dbl)
                }
                frame "s" {
                  n304 = Multiply(x=w729, y=1000000000.0) -> (x*y=w728:dbl)
                  n305 = Multiply(x=w728, y=3.0) -> (x*y=w731:dbl)
                }
              }
              n306 = Subtract(x=w706, y=w700) -> (x-y=w704:dbl)
              n307 = Divide(x=w704, y=2.0) -> (x/y=w703:dbl)
              n308 = Multiply(x=w707, y=w703) -> (x*y=w701:dbl)
              n309 = Multiply(x=w707, y=w705) -> (x*y=w708:dbl)
              n310 = Less?(x=w706, y=w705) -> (x < y?=w709:bool)
              n311 = Select(t=w701, s=w709, f=w708) -> (s? t:f=w697:dbl)
              n312 = Multiply(x=0.001, y=w697) -> (x*y=w698:dbl)
            }
            frame "us" {
              w744 = 0.795 ("lower limit")
              n313 = case shown="Default" w748 {
                tunnel: w747 -> [w749 w753 w758 w763 w768]
                tunnel: [w750 w755 w760 w765 w770] -> w742
                tunnel: [w749 w752 w757 w762 w767] -> w737
                frame Default {
                  n314 = Multiply(x=w749, y=3.0) -> (x*y=w750:dbl)
                }
                frame "ns" {
                  n315 = Multiply(x=w753, y=0.001) -> (x*y=w752:dbl)
                  n316 = Multiply(x=w752, y=3.0) -> (x*y=w755:dbl)
                }
                frame "us" {
                  n317 = Multiply(x=w758, y=1.0) -> (x*y=w757:dbl)
                  n318 = Multiply(x=w757, y=3.0) -> (x*y=w760:dbl)
                }
                frame "ms" {
                  n319 = Multiply(x=w763, y=1000.0) -> (x*y=w762:dbl)
                  n320 = Multiply(x=w762, y=3.0) -> (x*y=w765:dbl)
                }
                frame "s" {
                  n321 = Multiply(x=w768, y=1000000.0) -> (x*y=w767:dbl)
                  n322 = Multiply(x=w767, y=3.0) -> (x*y=w770:dbl)
                }
              }
              n323 = Subtract(x=w743, y=w737) -> (x-y=w741:dbl)
              n324 = Divide(x=w741, y=2.0) -> (x/y=w740:dbl)
              n325 = Multiply(x=w744, y=w740) -> (x*y=w738:dbl)
              n326 = Multiply(x=w744, y=w742) -> (x*y=w745:dbl)
              n327 = Less?(x=w743, y=w742) -> (x < y?=w746:bool)
              n328 = Select(t=w738, s=w746, f=w745) -> (s? t:f=w735:dbl)
              n329 = Multiply(x=1.0, y=w735) -> (x*y=w736:dbl)
            }
            frame "ms" {
              w783 = 0.795 ("lower limit")
              n330 = case shown="Default" w787 {
                tunnel: w786 -> [w788 w792 w797 w802 w807]
                tunnel: [w789 w794 w799 w804 w809] -> w781
                tunnel: [w788 w791 w796 w801 w806] -> w776
                frame Default {
                  n331 = Multiply(x=w788, y=3.0) -> (x*y=w789:dbl)
                }
                frame "ns" {
                  n332 = Multiply(x=w792, y=1e-06) -> (x*y=w791:dbl)
                  n333 = Multiply(x=w791, y=3.0) -> (x*y=w794:dbl)
                }
                frame "us" {
                  n334 = Multiply(x=w797, y=0.001) -> (x*y=w796:dbl)
                  n335 = Multiply(x=w796, y=3.0) -> (x*y=w799:dbl)
                }
                frame "ms" {
                  n336 = Multiply(x=w802, y=1.0) -> (x*y=w801:dbl)
                  n337 = Multiply(x=w801, y=3.0) -> (x*y=w804:dbl)
                }
                frame "s" {
                  n338 = Multiply(x=w807, y=1000.0) -> (x*y=w806:dbl)
                  n339 = Multiply(x=w806, y=3.0) -> (x*y=w809:dbl)
                }
              }
              n340 = Subtract(x=w782, y=w776) -> (x-y=w780:dbl)
              n341 = Divide(x=w780, y=2.0) -> (x/y=w779:dbl)
              n342 = Multiply(x=w783, y=w779) -> (x*y=w777:dbl)
              n343 = Multiply(x=w783, y=w781) -> (x*y=w784:dbl)
              n344 = Less?(x=w782, y=w781) -> (x < y?=w785:bool)
              n345 = Select(t=w777, s=w785, f=w784) -> (s? t:f=w774:dbl)
              n346 = Multiply(x=1000.0, y=w774) -> (x*y=w775:dbl)
            }
            frame "s" {
              w822 = 0.795 ("lower limit")
              n347 = case shown="Default" w826 {
                tunnel: w825 -> [w827 w831 w836 w841 w846]
                tunnel: [w828 w833 w838 w843 w848] -> w820
                tunnel: [w827 w830 w835 w840 w845] -> w815
                frame Default {
                  n348 = Multiply(x=w827, y=3.0) -> (x*y=w828:dbl)
                }
                frame "ns" {
                  n349 = Multiply(x=w831, y=1e-06) -> (x*y=w830:dbl)
                  n350 = Multiply(x=w830, y=3.0) -> (x*y=w833:dbl)
                }
                frame "us" {
                  n351 = Multiply(x=w836, y=0.001) -> (x*y=w835:dbl)
                  n352 = Multiply(x=w835, y=3.0) -> (x*y=w838:dbl)
                }
                frame "ms" {
                  n353 = Multiply(x=w841, y=1.0) -> (x*y=w840:dbl)
                  n354 = Multiply(x=w840, y=3.0) -> (x*y=w843:dbl)
                }
                frame "s" {
                  n355 = Multiply(x=w846, y=1000.0) -> (x*y=w845:dbl)
                  n356 = Multiply(x=w845, y=3.0) -> (x*y=w848:dbl)
                }
              }
              n357 = Subtract(x=w821, y=w815) -> (x-y=w819:dbl)
              n358 = Divide(x=w819, y=2.0) -> (x/y=w818:dbl)
              n359 = Multiply(x=w822, y=w818) -> (x*y=w816:dbl)
              n360 = Multiply(x=w822, y=w820) -> (x*y=w823:dbl)
              n361 = Less?(x=w821, y=w820) -> (x < y?=w824:bool)
              n362 = Select(t=w816, s=w824, f=w823) -> (s? t:f=w813:dbl)
              n363 = Multiply(x=1000000.0, y=w813) -> (x*y=w814:dbl)
            }
          }
          n364 = In Range and Coerce(upper limit=w681, x=w688, lower limit=10.0) -> (coerced(x)=w689:dbl, In Range?=w682:bool)
          n365 = case shown="False" w682 {
            tunnel: w681 -> [w691 _]
            tunnel: w680 -> [w690 _]
            frame False {
              n366 = Format Into String(format string="RisEdge time can`t be lower than 10 ns or higher than %.3f %s!" ("message"), w691, w690) -> (resulting string=w693:string)  [unwired: 2 in, 1 out]
              n367 = One Button Dialog(message=w693) -> ()  [unwired: 1 in, 1 out]
            }
            frame True {
            }
          }
        }
        frame "ms" {
          n368 = case shown="\"ns\"" w856 {
            tunnel: w855 -> [_ w876 w913 w952 w991]
            tunnel: w854 -> [w865 w880 w917 w956 w995]
            tunnel: w853 -> [_ w881 w918 w957 w996]
            tunnel: [w865 w868 w906 w945 w984] -> w851
            tunnel: ["ns" "ns" "us" "ms" "s"] -> w850
            frame Default {
            }
            frame "ns" {
              w877 = 0.795 ("lower limit")
              n369 = case shown="Default" w881 {
                tunnel: w880 -> [w882 w885 w889 w894 w899]
                tunnel: [w883 w886 w891 w896 w901] -> w875
                tunnel: [w882 w885 w888 w893 w898] -> w870
                frame Default {
                  n370 = Multiply(x=w882, y=3.0) -> (x*y=w883:dbl)
                }
                frame "ns" {
                  n371 = Multiply(x=w885, y=3.0) -> (x*y=w886:dbl)
                }
                frame "us" {
                  n372 = Multiply(x=w889, y=1000.0) -> (x*y=w888:dbl)
                  n373 = Multiply(x=w888, y=3.0) -> (x*y=w891:dbl)
                }
                frame "ms" {
                  n374 = Multiply(x=w894, y=1000000.0) -> (x*y=w893:dbl)
                  n375 = Multiply(x=w893, y=3.0) -> (x*y=w896:dbl)
                }
                frame "s" {
                  n376 = Multiply(x=w899, y=1000000000.0) -> (x*y=w898:dbl)
                  n377 = Multiply(x=w898, y=3.0) -> (x*y=w901:dbl)
                }
              }
              n378 = Subtract(x=w876, y=w870) -> (x-y=w874:dbl)
              n379 = Divide(x=w874, y=2.0) -> (x/y=w873:dbl)
              n380 = Multiply(x=w877, y=w873) -> (x*y=w871:dbl)
              n381 = Multiply(x=w877, y=w875) -> (x*y=w878:dbl)
              n382 = Less?(x=w876, y=w875) -> (x < y?=w879:bool)
              n383 = Select(t=w871, s=w879, f=w878) -> (s? t:f=w867:dbl)
              n384 = Multiply(x=1e-06, y=w867) -> (x*y=w868:dbl)
            }
            frame "us" {
              w914 = 0.795 ("lower limit")
              n385 = case shown="Default" w918 {
                tunnel: w917 -> [w919 w923 w928 w933 w938]
                tunnel: [w920 w925 w930 w935 w940] -> w912
                tunnel: [w919 w922 w927 w932 w937] -> w907
                frame Default {
                  n386 = Multiply(x=w919, y=3.0) -> (x*y=w920:dbl)
                }
                frame "ns" {
                  n387 = Multiply(x=w923, y=0.001) -> (x*y=w922:dbl)
                  n388 = Multiply(x=w922, y=3.0) -> (x*y=w925:dbl)
                }
                frame "us" {
                  n389 = Multiply(x=w928, y=1.0) -> (x*y=w927:dbl)
                  n390 = Multiply(x=w927, y=3.0) -> (x*y=w930:dbl)
                }
                frame "ms" {
                  n391 = Multiply(x=w933, y=1000.0) -> (x*y=w932:dbl)
                  n392 = Multiply(x=w932, y=3.0) -> (x*y=w935:dbl)
                }
                frame "s" {
                  n393 = Multiply(x=w938, y=1000000.0) -> (x*y=w937:dbl)
                  n394 = Multiply(x=w937, y=3.0) -> (x*y=w940:dbl)
                }
              }
              n395 = Subtract(x=w913, y=w907) -> (x-y=w911:dbl)
              n396 = Divide(x=w911, y=2.0) -> (x/y=w910:dbl)
              n397 = Multiply(x=w914, y=w910) -> (x*y=w908:dbl)
              n398 = Multiply(x=w914, y=w912) -> (x*y=w915:dbl)
              n399 = Less?(x=w913, y=w912) -> (x < y?=w916:bool)
              n400 = Select(t=w908, s=w916, f=w915) -> (s? t:f=w905:dbl)
              n401 = Multiply(x=0.001, y=w905) -> (x*y=w906:dbl)
            }
            frame "ms" {
              w953 = 0.795 ("lower limit")
              n402 = case shown="Default" w957 {
                tunnel: w956 -> [w958 w962 w967 w972 w977]
                tunnel: [w959 w964 w969 w974 w979] -> w951
                tunnel: [w958 w961 w966 w971 w976] -> w946
                frame Default {
                  n403 = Multiply(x=w958, y=3.0) -> (x*y=w959:dbl)
                }
                frame "ns" {
                  n404 = Multiply(x=w962, y=1e-06) -> (x*y=w961:dbl)
                  n405 = Multiply(x=w961, y=3.0) -> (x*y=w964:dbl)
                }
                frame "us" {
                  n406 = Multiply(x=w967, y=0.001) -> (x*y=w966:dbl)
                  n407 = Multiply(x=w966, y=3.0) -> (x*y=w969:dbl)
                }
                frame "ms" {
                  n408 = Multiply(x=w972, y=1.0) -> (x*y=w971:dbl)
                  n409 = Multiply(x=w971, y=3.0) -> (x*y=w974:dbl)
                }
                frame "s" {
                  n410 = Multiply(x=w977, y=1000.0) -> (x*y=w976:dbl)
                  n411 = Multiply(x=w976, y=3.0) -> (x*y=w979:dbl)
                }
              }
              n412 = Subtract(x=w952, y=w946) -> (x-y=w950:dbl)
              n413 = Divide(x=w950, y=2.0) -> (x/y=w949:dbl)
              n414 = Multiply(x=w953, y=w949) -> (x*y=w947:dbl)
              n415 = Multiply(x=w953, y=w951) -> (x*y=w954:dbl)
              n416 = Less?(x=w952, y=w951) -> (x < y?=w955:bool)
              n417 = Select(t=w947, s=w955, f=w954) -> (s? t:f=w944:dbl)
              n418 = Multiply(x=1.0, y=w944) -> (x*y=w945:dbl)
            }
            frame "s" {
              w992 = 0.795 ("lower limit")
              n419 = case shown="Default" w996 {
                tunnel: w995 -> [w997 w1001 w1006 w1011 w1016]
                tunnel: [w998 w1003 w1008 w1013 w1018] -> w990
                tunnel: [w997 w1000 w1005 w1010 w1015] -> w985
                frame Default {
                  n420 = Multiply(x=w997, y=3.0) -> (x*y=w998:dbl)
                }
                frame "ns" {
                  n421 = Multiply(x=w1001, y=1e-06) -> (x*y=w1000:dbl)
                  n422 = Multiply(x=w1000, y=3.0) -> (x*y=w1003:dbl)
                }
                frame "us" {
                  n423 = Multiply(x=w1006, y=0.001) -> (x*y=w1005:dbl)
                  n424 = Multiply(x=w1005, y=3.0) -> (x*y=w1008:dbl)
                }
                frame "ms" {
                  n425 = Multiply(x=w1011, y=1.0) -> (x*y=w1010:dbl)
                  n426 = Multiply(x=w1010, y=3.0) -> (x*y=w1013:dbl)
                }
                frame "s" {
                  n427 = Multiply(x=w1016, y=1000.0) -> (x*y=w1015:dbl)
                  n428 = Multiply(x=w1015, y=3.0) -> (x*y=w1018:dbl)
                }
              }
              n429 = Subtract(x=w991, y=w985) -> (x-y=w989:dbl)
              n430 = Divide(x=w989, y=2.0) -> (x/y=w988:dbl)
              n431 = Multiply(x=w992, y=w988) -> (x*y=w986:dbl)
              n432 = Multiply(x=w992, y=w990) -> (x*y=w993:dbl)
              n433 = Less?(x=w991, y=w990) -> (x < y?=w994:bool)
              n434 = Select(t=w986, s=w994, f=w993) -> (s? t:f=w983:dbl)
              n435 = Multiply(x=1000.0, y=w983) -> (x*y=w984:dbl)
            }
          }
          n436 = In Range and Coerce(upper limit=w851, x=w858, lower limit=10.0) -> (coerced(x)=w859:dbl, In Range?=w852:bool)
          n437 = case shown="False" w852 {
            tunnel: w851 -> [w861 _]
            tunnel: w850 -> [w860 _]
            frame False {
              n438 = Format Into String(format string="RisEdge time can`t be lower than 10 ns or higher than %.3f %s!" ("message"), w861, w860) -> (resulting string=w863:string)  [unwired: 2 in, 1 out]
              n439 = One Button Dialog(message=w863) -> ()  [unwired: 1 in, 1 out]
            }
            frame True {
            }
          }
        }
        frame "s" {
          n440 = case shown="Default" w1026 {
            tunnel: w1025 -> [_ w1046 w1083 w1122 w1161]
            tunnel: w1024 -> [w1035 w1050 w1087 w1126 w1165]
            tunnel: w1023 -> [_ w1051 w1088 w1127 w1166]
            tunnel: [w1035 w1038 w1076 w1115 w1154] -> w1021
            tunnel: ["ns" "ns" "us" "ms" "s"] -> w1020
            frame Default {
            }
            frame "ns" {
              w1047 = 0.795 ("lower limit")
              n441 = case shown="Default" w1051 {
                tunnel: w1050 -> [w1052 w1055 w1059 w1064 w1069]
                tunnel: [w1053 w1056 w1061 w1066 w1071] -> w1045
                tunnel: [w1052 w1055 w1058 w1063 w1068] -> w1040
                frame Default {
                  n442 = Multiply(x=w1052, y=3.0) -> (x*y=w1053:dbl)
                }
                frame "ns" {
                  n443 = Multiply(x=w1055, y=3.0) -> (x*y=w1056:dbl)
                }
                frame "us" {
                  n444 = Multiply(x=w1059, y=1000.0) -> (x*y=w1058:dbl)
                  n445 = Multiply(x=w1058, y=3.0) -> (x*y=w1061:dbl)
                }
                frame "ms" {
                  n446 = Multiply(x=w1064, y=1000000.0) -> (x*y=w1063:dbl)
                  n447 = Multiply(x=w1063, y=3.0) -> (x*y=w1066:dbl)
                }
                frame "s" {
                  n448 = Multiply(x=w1069, y=1000000000.0) -> (x*y=w1068:dbl)
                  n449 = Multiply(x=w1068, y=3.0) -> (x*y=w1071:dbl)
                }
              }
              n450 = Subtract(x=w1046, y=w1040) -> (x-y=w1044:dbl)
              n451 = Divide(x=w1044, y=2.0) -> (x/y=w1043:dbl)
              n452 = Multiply(x=w1047, y=w1043) -> (x*y=w1041:dbl)
              n453 = Multiply(x=w1047, y=w1045) -> (x*y=w1048:dbl)
              n454 = Less?(x=w1046, y=w1045) -> (x < y?=w1049:bool)
              n455 = Select(t=w1041, s=w1049, f=w1048) -> (s? t:f=w1037:dbl)
              n456 = Multiply(x=1e-09, y=w1037) -> (x*y=w1038:dbl)
            }
            frame "us" {
              w1084 = 0.795 ("lower limit")
              n457 = case shown="Default" w1088 {
                tunnel: w1087 -> [w1089 w1093 w1098 w1103 w1108]
                tunnel: [w1090 w1095 w1100 w1105 w1110] -> w1082
                tunnel: [w1089 w1092 w1097 w1102 w1107] -> w1077
                frame Default {
                  n458 = Multiply(x=w1089, y=3.0) -> (x*y=w1090:dbl)
                }
                frame "ns" {
                  n459 = Multiply(x=w1093, y=0.001) -> (x*y=w1092:dbl)
                  n460 = Multiply(x=w1092, y=3.0) -> (x*y=w1095:dbl)
                }
                frame "us" {
                  n461 = Multiply(x=w1098, y=1.0) -> (x*y=w1097:dbl)
                  n462 = Multiply(x=w1097, y=3.0) -> (x*y=w1100:dbl)
                }
                frame "ms" {
                  n463 = Multiply(x=w1103, y=1000.0) -> (x*y=w1102:dbl)
                  n464 = Multiply(x=w1102, y=3.0) -> (x*y=w1105:dbl)
                }
                frame "s" {
                  n465 = Multiply(x=w1108, y=1000000.0) -> (x*y=w1107:dbl)
                  n466 = Multiply(x=w1107, y=3.0) -> (x*y=w1110:dbl)
                }
              }
              n467 = Subtract(x=w1083, y=w1077) -> (x-y=w1081:dbl)
              n468 = Divide(x=w1081, y=2.0) -> (x/y=w1080:dbl)
              n469 = Multiply(x=w1084, y=w1080) -> (x*y=w1078:dbl)
              n470 = Multiply(x=w1084, y=w1082) -> (x*y=w1085:dbl)
              n471 = Less?(x=w1083, y=w1082) -> (x < y?=w1086:bool)
              n472 = Select(t=w1078, s=w1086, f=w1085) -> (s? t:f=w1075:dbl)
              n473 = Multiply(x=1e-06, y=w1075) -> (x*y=w1076:dbl)
            }
            frame "ms" {
              w1123 = 0.795 ("lower limit")
              n474 = case shown="Default" w1127 {
                tunnel: w1126 -> [w1128 w1132 w1137 w1142 w1147]
                tunnel: [w1129 w1134 w1139 w1144 w1149] -> w1121
                tunnel: [w1128 w1131 w1136 w1141 w1146] -> w1116
                frame Default {
                  n475 = Multiply(x=w1128, y=3.0) -> (x*y=w1129:dbl)
                }
                frame "ns" {
                  n476 = Multiply(x=w1132, y=1e-06) -> (x*y=w1131:dbl)
                  n477 = Multiply(x=w1131, y=3.0) -> (x*y=w1134:dbl)
                }
                frame "us" {
                  n478 = Multiply(x=w1137, y=0.001) -> (x*y=w1136:dbl)
                  n479 = Multiply(x=w1136, y=3.0) -> (x*y=w1139:dbl)
                }
                frame "ms" {
                  n480 = Multiply(x=w1142, y=1.0) -> (x*y=w1141:dbl)
                  n481 = Multiply(x=w1141, y=3.0) -> (x*y=w1144:dbl)
                }
                frame "s" {
                  n482 = Multiply(x=w1147, y=1000.0) -> (x*y=w1146:dbl)
                  n483 = Multiply(x=w1146, y=3.0) -> (x*y=w1149:dbl)
                }
              }
              n484 = Subtract(x=w1122, y=w1116) -> (x-y=w1120:dbl)
              n485 = Divide(x=w1120, y=2.0) -> (x/y=w1119:dbl)
              n486 = Multiply(x=w1123, y=w1119) -> (x*y=w1117:dbl)
              n487 = Multiply(x=w1123, y=w1121) -> (x*y=w1124:dbl)
              n488 = Less?(x=w1122, y=w1121) -> (x < y?=w1125:bool)
              n489 = Select(t=w1117, s=w1125, f=w1124) -> (s? t:f=w1114:dbl)
              n490 = Multiply(x=0.001, y=w1114) -> (x*y=w1115:dbl)
            }
            frame "s" {
              w1162 = 0.795 ("lower limit")
              n491 = case shown="Default" w1166 {
                tunnel: w1165 -> [w1167 w1171 w1176 w1181 w1186]
                tunnel: [w1168 w1173 w1178 w1183 w1188] -> w1160
                tunnel: [w1167 w1170 w1175 w1180 w1185] -> w1155
                frame Default {
                  n492 = Multiply(x=w1167, y=3.0) -> (x*y=w1168:dbl)
                }
                frame "ns" {
                  n493 = Multiply(x=w1171, y=1e-06) -> (x*y=w1170:dbl)
                  n494 = Multiply(x=w1170, y=3.0) -> (x*y=w1173:dbl)
                }
                frame "us" {
                  n495 = Multiply(x=w1176, y=0.001) -> (x*y=w1175:dbl)
                  n496 = Multiply(x=w1175, y=3.0) -> (x*y=w1178:dbl)
                }
                frame "ms" {
                  n497 = Multiply(x=w1181, y=1.0) -> (x*y=w1180:dbl)
                  n498 = Multiply(x=w1180, y=3.0) -> (x*y=w1183:dbl)
                }
                frame "s" {
                  n499 = Multiply(x=w1186, y=1000.0) -> (x*y=w1185:dbl)
                  n500 = Multiply(x=w1185, y=3.0) -> (x*y=w1188:dbl)
                }
              }
              n501 = Subtract(x=w1161, y=w1155) -> (x-y=w1159:dbl)
              n502 = Divide(x=w1159, y=2.0) -> (x/y=w1158:dbl)
              n503 = Multiply(x=w1162, y=w1158) -> (x*y=w1156:dbl)
              n504 = Multiply(x=w1162, y=w1160) -> (x*y=w1163:dbl)
              n505 = Less?(x=w1161, y=w1160) -> (x < y?=w1164:bool)
              n506 = Select(t=w1156, s=w1164, f=w1163) -> (s? t:f=w1153:dbl)
              n507 = Multiply(x=1.0, y=w1153) -> (x*y=w1154:dbl)
            }
          }
          n508 = In Range and Coerce(upper limit=w1021, x=w1028, lower limit=10.0) -> (coerced(x)=w1029:dbl, In Range?=w1022:bool)
          n509 = case shown="False" w1022 {
            tunnel: w1021 -> [w1031 _]
            tunnel: w1020 -> [w1030 _]
            frame False {
              n510 = Format Into String(format string="RisEdge time can`t be lower than 10 ns or higher than %.3f %s!" ("message"), w1031, w1030) -> (resulting string=w1033:string)  [unwired: 2 in, 1 out]
              n511 = One Button Dialog(message=w1033) -> ()  [unwired: 1 in, 1 out]
            }
            frame True {
            }
          }
        }
      }
      n512 = Bundle By Name(cluster=w508, "RisEdge"=w499) -> (w505:T13)
      n513 = To Variant(anything=w505) -> (Variant=w504:variant)
    }
    frame "FallEdge" {
      n514 = Variant To Data(error in=w1202, type=T14 {"FallEdge"=10.0, "FallEdgeUnit"=enum."ns", "FallEdgeUnitPrcs"=1.0} ("FallEdge"), Variant=w1204) -> (data=w1203:T14, error out=w1201:errorcluster)
      n515 = Unbundle By Name(w1203) -> ("FallEdge"=w1197:dbl, "FallEdgeUnit"=w1196:enum32{"No Selection", "s", "ms", "us", "ns"})
      n516 = Unbundle By Name(w1198) -> ("Period"=w1193:dbl, "PeriodUnit"=w1194:enum32{"No Selection", "s", "ms", "us", "ns"}, "Width"=w1192:dbl, "WidthUnit"=w1191:enum32{"No Selection", "s", "ms", "us", "ns"})
      n517 = case shown="\"ms\"" w1196 {
        tunnel: w1197 -> [w1205 w1215 w1383 w1553 w1723]
        tunnel: [w1205 w1216 w1384 w1554 w1724] -> w1195
        tunnel: w1194 -> [_ w1213 w1381 w1551 w1721]
        tunnel: w1193 -> [_ w1212 w1380 w1550 w1720]
        tunnel: w1192 -> [_ w1211 w1379 w1549 w1719]
        tunnel: w1191 -> [_ w1210 w1378 w1548 w1718]
        frame Default {
        }
        frame "ns" {
          n518 = case shown="\"s\"" w1213 {
            tunnel: w1212 -> [_ w1231 w1268 w1307 w1346]
            tunnel: w1211 -> [w1221 w1235 w1272 w1311 w1350]
            tunnel: w1210 -> [_ w1236 w1273 w1312 w1351]
            tunnel: [w1221 w1223 w1261 w1300 w1339] -> w1207
            tunnel: ["ns" "ns" "us" "ms" "s"] -> w1209
            tunnel: [w1221 w1223 w1258 w1297 w1336] -> w1206
            frame Default {
            }
            frame "ns" {
              w1232 = 0.795 ("lower limit")
              n519 = case shown="\"ns\"" w1236 {
                tunnel: w1235 -> [w1238 w1240 w1244 w1249 w1254]
                tunnel: [w1239 w1241 w1246 w1251 w1256] -> w1230
                tunnel: [w1238 w1240 w1243 w1248 w1253] -> w1225
                frame Default {
                  n520 = Multiply(x=w1238, y=3.0) -> (x*y=w1239:dbl)
                }
                frame "ns" {
                  n521 = Multiply(x=w1240, y=3.0) -> (x*y=w1241:dbl)
                }
                frame "us" {
                  n522 = Multiply(x=w1244, y=1000.0) -> (x*y=w1243:dbl)
                  n523 = Multiply(x=w1243, y=3.0) -> (x*y=w1246:dbl)
                }
                frame "ms" {
                  n524 = Multiply(x=w1249, y=1000000.0) -> (x*y=w1248:dbl)
                  n525 = Multiply(x=w1248, y=3.0) -> (x*y=w1251:dbl)
                }
                frame "s" {
                  n526 = Multiply(x=w1254, y=1000000000.0) -> (x*y=w1253:dbl)
                  n527 = Multiply(x=w1253, y=3.0) -> (x*y=w1256:dbl)
                }
              }
              n528 = Subtract(x=w1231, y=w1225) -> (x-y=w1229:dbl)
              n529 = Divide(x=w1229, y=2.0) -> (x/y=w1228:dbl)
              n530 = Multiply(x=w1232, y=w1228) -> (x*y=w1226:dbl)
              n531 = Multiply(x=w1232, y=w1230) -> (x*y=w1233:dbl)
              n532 = Less?(x=w1231, y=w1230) -> (x < y?=w1234:bool)
              n533 = Select(t=w1226, s=w1234, f=w1233) -> (s? t:f=w1223:dbl)
            }
            frame "us" {
              w1269 = 0.795 ("lower limit")
              n534 = case shown="Default" w1273 {
                tunnel: w1272 -> [w1274 w1278 w1283 w1288 w1293]
                tunnel: [w1275 w1280 w1285 w1290 w1295] -> w1267
                tunnel: [w1274 w1277 w1282 w1287 w1292] -> w1262
                frame Default {
                  n535 = Multiply(x=w1274, y=3.0) -> (x*y=w1275:dbl)
                }
                frame "ns" {
                  n536 = Multiply(x=w1278, y=0.001) -> (x*y=w1277:dbl)
                  n537 = Multiply(x=w1277, y=3.0) -> (x*y=w1280:dbl)
                }
                frame "us" {
                  n538 = Multiply(x=w1283, y=1.0) -> (x*y=w1282:dbl)
                  n539 = Multiply(x=w1282, y=3.0) -> (x*y=w1285:dbl)
                }
                frame "ms" {
                  n540 = Multiply(x=w1288, y=1000.0) -> (x*y=w1287:dbl)
                  n541 = Multiply(x=w1287, y=3.0) -> (x*y=w1290:dbl)
                }
                frame "s" {
                  n542 = Multiply(x=w1293, y=1000000.0) -> (x*y=w1292:dbl)
                  n543 = Multiply(x=w1292, y=3.0) -> (x*y=w1295:dbl)
                }
              }
              n544 = Subtract(x=w1268, y=w1262) -> (x-y=w1266:dbl)
              n545 = Divide(x=w1266, y=2.0) -> (x/y=w1265:dbl)
              n546 = Multiply(x=w1269, y=w1265) -> (x*y=w1263:dbl)
              n547 = Multiply(x=w1269, y=w1267) -> (x*y=w1270:dbl)
              n548 = Less?(x=w1268, y=w1267) -> (x < y?=w1271:bool)
              n549 = Select(t=w1263, s=w1271, f=w1270) -> (s? t:f=w1258:dbl)
              n550 = Multiply(x=1000.0, y=w1258) -> (x*y=w1261:dbl)
            }
            frame "ms" {
              w1308 = 0.795 ("lower limit")
              n551 = case shown="\"us\"" w1312 {
                tunnel: w1311 -> [w1313 w1317 w1322 w1327 w1332]
                tunnel: [w1314 w1319 w1324 w1329 w1334] -> w1306
                tunnel: [w1313 w1316 w1321 w1326 w1331] -> w1301
                frame Default {
                  n552 = Multiply(x=w1313, y=3.0) -> (x*y=w1314:dbl)
                }
                frame "ns" {
                  n553 = Multiply(x=w1317, y=1e-06) -> (x*y=w1316:dbl)
                  n554 = Multiply(x=w1316, y=3.0) -> (x*y=w1319:dbl)
                }
                frame "us" {
                  n555 = Multiply(x=w1322, y=0.001) -> (x*y=w1321:dbl)
                  n556 = Multiply(x=w1321, y=3.0) -> (x*y=w1324:dbl)
                }
                frame "ms" {
                  n557 = Multiply(x=w1327, y=1.0) -> (x*y=w1326:dbl)
                  n558 = Multiply(x=w1326, y=3.0) -> (x*y=w1329:dbl)
                }
                frame "s" {
                  n559 = Multiply(x=w1332, y=1000.0) -> (x*y=w1331:dbl)
                  n560 = Multiply(x=w1331, y=3.0) -> (x*y=w1334:dbl)
                }
              }
              n561 = Subtract(x=w1307, y=w1301) -> (x-y=w1305:dbl)
              n562 = Divide(x=w1305, y=2.0) -> (x/y=w1304:dbl)
              n563 = Multiply(x=w1308, y=w1304) -> (x*y=w1302:dbl)
              n564 = Multiply(x=w1308, y=w1306) -> (x*y=w1309:dbl)
              n565 = Less?(x=w1307, y=w1306) -> (x < y?=w1310:bool)
              n566 = Select(t=w1302, s=w1310, f=w1309) -> (s? t:f=w1297:dbl)
              n567 = Multiply(x=1000000.0, y=w1297) -> (x*y=w1300:dbl)
            }
            frame "s" {
              w1347 = 0.795 ("lower limit")
              n568 = case shown="\"ns\"" w1351 {
                tunnel: w1350 -> [w1353 w1356 w1361 w1366 w1371]
                tunnel: [w1352 w1358 w1363 w1368 w1373] -> w1345
                tunnel: [w1353 w1355 w1360 w1365 w1370] -> w1340
                frame Default {
                  n569 = Multiply(x=w1353, y=3.0) -> (x*y=w1352:dbl)
                }
                frame "ns" {
                  n570 = Multiply(x=w1356, y=1e-06) -> (x*y=w1355:dbl)
                  n571 = Multiply(x=w1355, y=3.0) -> (x*y=w1358:dbl)
                }
                frame "us" {
                  n572 = Multiply(x=w1361, y=0.001) -> (x*y=w1360:dbl)
                  n573 = Multiply(x=w1360, y=3.0) -> (x*y=w1363:dbl)
                }
                frame "ms" {
                  n574 = Multiply(x=w1366, y=1.0) -> (x*y=w1365:dbl)
                  n575 = Multiply(x=w1365, y=3.0) -> (x*y=w1368:dbl)
                }
                frame "s" {
                  n576 = Multiply(x=w1371, y=1000.0) -> (x*y=w1370:dbl)
                  n577 = Multiply(x=w1370, y=3.0) -> (x*y=w1373:dbl)
                }
              }
              n578 = Subtract(x=w1346, y=w1340) -> (x-y=w1344:dbl)
              n579 = Divide(x=w1344, y=2.0) -> (x/y=w1343:dbl)
              n580 = Multiply(x=w1347, y=w1343) -> (x*y=w1341:dbl)
              n581 = Multiply(x=w1347, y=w1345) -> (x*y=w1348:dbl)
              n582 = Less?(x=w1346, y=w1345) -> (x < y?=w1349:bool)
              n583 = Select(t=w1341, s=w1349, f=w1348) -> (s? t:f=w1336:dbl)
              n584 = Multiply(x=1000000000.0, y=w1336) -> (x*y=w1339:dbl)
            }
          }
          n585 = In Range and Coerce(upper limit=w1207, x=w1215, lower limit=10.0) -> (coerced(x)=w1216:dbl, In Range?=w1208:bool)
          n586 = case shown="False" w1208 {
            tunnel: w1206 -> [w1218 _]
            tunnel: w1209 -> [w1217 _]
            frame False {
              n587 = Format Into String(format string="FallEdge time can`t be lower than 10 ns or higher than %.3f %s!" ("message"), w1218, w1217) -> (resulting string=w1220:string)  [unwired: 2 in, 1 out]
              n588 = One Button Dialog(message=w1220) -> ()  [unwired: 1 in, 1 out]
            }
            frame True {
            }
          }
        }
        frame "us" {
          n589 = case shown="\"ns\"" w1381 {
            tunnel: w1380 -> [_ w1401 w1438 w1477 w1516]
            tunnel: w1379 -> [w1390 w1405 w1442 w1481 w1520]
            tunnel: w1378 -> [_ w1406 w1443 w1482 w1521]
            tunnel: [w1390 w1393 w1431 w1470 w1509] -> w1376
            tunnel: ["ns" "ns" "us" "ms" "s"] -> w1375
            frame Default {
            }
            frame "ns" {
              w1402 = 0.795 ("lower limit")
              n590 = case shown="Default" w1406 {
                tunnel: w1405 -> [w1407 w1410 w1414 w1419 w1424]
                tunnel: [w1408 w1411 w1416 w1421 w1426] -> w1400
                tunnel: [w1407 w1410 w1413 w1418 w1423] -> w1395
                frame Default {
                  n591 = Multiply(x=w1407, y=3.0) -> (x*y=w1408:dbl)
                }
                frame "ns" {
                  n592 = Multiply(x=w1410, y=3.0) -> (x*y=w1411:dbl)
                }
                frame "us" {
                  n593 = Multiply(x=w1414, y=1000.0) -> (x*y=w1413:dbl)
                  n594 = Multiply(x=w1413, y=3.0) -> (x*y=w1416:dbl)
                }
                frame "ms" {
                  n595 = Multiply(x=w1419, y=1000000.0) -> (x*y=w1418:dbl)
                  n596 = Multiply(x=w1418, y=3.0) -> (x*y=w1421:dbl)
                }
                frame "s" {
                  n597 = Multiply(x=w1424, y=1000000000.0) -> (x*y=w1423:dbl)
                  n598 = Multiply(x=w1423, y=3.0) -> (x*y=w1426:dbl)
                }
              }
              n599 = Subtract(x=w1401, y=w1395) -> (x-y=w1399:dbl)
              n600 = Divide(x=w1399, y=2.0) -> (x/y=w1398:dbl)
              n601 = Multiply(x=w1402, y=w1398) -> (x*y=w1396:dbl)
              n602 = Multiply(x=w1402, y=w1400) -> (x*y=w1403:dbl)
              n603 = Less?(x=w1401, y=w1400) -> (x < y?=w1404:bool)
              n604 = Select(t=w1396, s=w1404, f=w1403) -> (s? t:f=w1392:dbl)
              n605 = Multiply(x=0.001, y=w1392) -> (x*y=w1393:dbl)
            }
            frame "us" {
              w1439 = 0.795 ("lower limit")
              n606 = case shown="Default" w1443 {
                tunnel: w1442 -> [w1444 w1448 w1453 w1458 w1463]
                tunnel: [w1445 w1450 w1455 w1460 w1465] -> w1437
                tunnel: [w1444 w1447 w1452 w1457 w1462] -> w1432
                frame Default {
                  n607 = Multiply(x=w1444, y=3.0) -> (x*y=w1445:dbl)
                }
                frame "ns" {
                  n608 = Multiply(x=w1448, y=0.001) -> (x*y=w1447:dbl)
                  n609 = Multiply(x=w1447, y=3.0) -> (x*y=w1450:dbl)
                }
                frame "us" {
                  n610 = Multiply(x=w1453, y=1.0) -> (x*y=w1452:dbl)
                  n611 = Multiply(x=w1452, y=3.0) -> (x*y=w1455:dbl)
                }
                frame "ms" {
                  n612 = Multiply(x=w1458, y=1000.0) -> (x*y=w1457:dbl)
                  n613 = Multiply(x=w1457, y=3.0) -> (x*y=w1460:dbl)
                }
                frame "s" {
                  n614 = Multiply(x=w1463, y=1000000.0) -> (x*y=w1462:dbl)
                  n615 = Multiply(x=w1462, y=3.0) -> (x*y=w1465:dbl)
                }
              }
              n616 = Subtract(x=w1438, y=w1432) -> (x-y=w1436:dbl)
              n617 = Divide(x=w1436, y=2.0) -> (x/y=w1435:dbl)
              n618 = Multiply(x=w1439, y=w1435) -> (x*y=w1433:dbl)
              n619 = Multiply(x=w1439, y=w1437) -> (x*y=w1440:dbl)
              n620 = Less?(x=w1438, y=w1437) -> (x < y?=w1441:bool)
              n621 = Select(t=w1433, s=w1441, f=w1440) -> (s? t:f=w1430:dbl)
              n622 = Multiply(x=1.0, y=w1430) -> (x*y=w1431:dbl)
            }
            frame "ms" {
              w1478 = 0.795 ("lower limit")
              n623 = case shown="Default" w1482 {
                tunnel: w1481 -> [w1483 w1487 w1492 w1497 w1502]
                tunnel: [w1484 w1489 w1494 w1499 w1504] -> w1476
                tunnel: [w1483 w1486 w1491 w1496 w1501] -> w1471
                frame Default {
                  n624 = Multiply(x=w1483, y=3.0) -> (x*y=w1484:dbl)
                }
                frame "ns" {
                  n625 = Multiply(x=w1487, y=1e-06) -> (x*y=w1486:dbl)
                  n626 = Multiply(x=w1486, y=3.0) -> (x*y=w1489:dbl)
                }
                frame "us" {
                  n627 = Multiply(x=w1492, y=0.001) -> (x*y=w1491:dbl)
                  n628 = Multiply(x=w1491, y=3.0) -> (x*y=w1494:dbl)
                }
                frame "ms" {
                  n629 = Multiply(x=w1497, y=1.0) -> (x*y=w1496:dbl)
                  n630 = Multiply(x=w1496, y=3.0) -> (x*y=w1499:dbl)
                }
                frame "s" {
                  n631 = Multiply(x=w1502, y=1000.0) -> (x*y=w1501:dbl)
                  n632 = Multiply(x=w1501, y=3.0) -> (x*y=w1504:dbl)
                }
              }
              n633 = Subtract(x=w1477, y=w1471) -> (x-y=w1475:dbl)
              n634 = Divide(x=w1475, y=2.0) -> (x/y=w1474:dbl)
              n635 = Multiply(x=w1478, y=w1474) -> (x*y=w1472:dbl)
              n636 = Multiply(x=w1478, y=w1476) -> (x*y=w1479:dbl)
              n637 = Less?(x=w1477, y=w1476) -> (x < y?=w1480:bool)
              n638 = Select(t=w1472, s=w1480, f=w1479) -> (s? t:f=w1469:dbl)
              n639 = Multiply(x=1000.0, y=w1469) -> (x*y=w1470:dbl)
            }
            frame "s" {
              w1517 = 0.795 ("lower limit")
              n640 = case shown="Default" w1521 {
                tunnel: w1520 -> [w1522 w1526 w1531 w1536 w1541]
                tunnel: [w1523 w1528 w1533 w1538 w1543] -> w1515
                tunnel: [w1522 w1525 w1530 w1535 w1540] -> w1510
                frame Default {
                  n641 = Multiply(x=w1522, y=3.0) -> (x*y=w1523:dbl)
                }
                frame "ns" {
                  n642 = Multiply(x=w1526, y=1e-06) -> (x*y=w1525:dbl)
                  n643 = Multiply(x=w1525, y=3.0) -> (x*y=w1528:dbl)
                }
                frame "us" {
                  n644 = Multiply(x=w1531, y=0.001) -> (x*y=w1530:dbl)
                  n645 = Multiply(x=w1530, y=3.0) -> (x*y=w1533:dbl)
                }
                frame "ms" {
                  n646 = Multiply(x=w1536, y=1.0) -> (x*y=w1535:dbl)
                  n647 = Multiply(x=w1535, y=3.0) -> (x*y=w1538:dbl)
                }
                frame "s" {
                  n648 = Multiply(x=w1541, y=1000.0) -> (x*y=w1540:dbl)
                  n649 = Multiply(x=w1540, y=3.0) -> (x*y=w1543:dbl)
                }
              }
              n650 = Subtract(x=w1516, y=w1510) -> (x-y=w1514:dbl)
              n651 = Divide(x=w1514, y=2.0) -> (x/y=w1513:dbl)
              n652 = Multiply(x=w1517, y=w1513) -> (x*y=w1511:dbl)
              n653 = Multiply(x=w1517, y=w1515) -> (x*y=w1518:dbl)
              n654 = Less?(x=w1516, y=w1515) -> (x < y?=w1519:bool)
              n655 = Select(t=w1511, s=w1519, f=w1518) -> (s? t:f=w1508:dbl)
              n656 = Multiply(x=1000000.0, y=w1508) -> (x*y=w1509:dbl)
            }
          }
          n657 = In Range and Coerce(upper limit=w1376, x=w1383, lower limit=10.0) -> (coerced(x)=w1384:dbl, In Range?=w1377:bool)
          n658 = case shown="False" w1377 {
            tunnel: w1376 -> [w1386 _]
            tunnel: w1375 -> [w1385 _]
            frame False {
              n659 = Format Into String(format string="FallEdge time can`t be lower than 10 ns or higher than %.3f %s!" ("message"), w1386, w1385) -> (resulting string=w1388:string)  [unwired: 2 in, 1 out]
              n660 = One Button Dialog(message=w1388) -> ()  [unwired: 1 in, 1 out]
            }
            frame True {
            }
          }
        }
        frame "ms" {
          n661 = case shown="\"ns\"" w1551 {
            tunnel: w1550 -> [_ w1571 w1608 w1647 w1686]
            tunnel: w1549 -> [w1560 w1575 w1612 w1651 w1690]
            tunnel: w1548 -> [_ w1576 w1613 w1652 w1691]
            tunnel: [w1560 w1563 w1601 w1640 w1679] -> w1546
            tunnel: ["ns" "ns" "us" "ms" "s"] -> w1545
            frame Default {
            }
            frame "ns" {
              w1572 = 0.795 ("lower limit")
              n662 = case shown="Default" w1576 {
                tunnel: w1575 -> [w1577 w1580 w1584 w1589 w1594]
                tunnel: [w1578 w1581 w1586 w1591 w1596] -> w1570
                tunnel: [w1577 w1580 w1583 w1588 w1593] -> w1565
                frame Default {
                  n663 = Multiply(x=w1577, y=3.0) -> (x*y=w1578:dbl)
                }
                frame "ns" {
                  n664 = Multiply(x=w1580, y=3.0) -> (x*y=w1581:dbl)
                }
                frame "us" {
                  n665 = Multiply(x=w1584, y=1000.0) -> (x*y=w1583:dbl)
                  n666 = Multiply(x=w1583, y=3.0) -> (x*y=w1586:dbl)
                }
                frame "ms" {
                  n667 = Multiply(x=w1589, y=1000000.0) -> (x*y=w1588:dbl)
                  n668 = Multiply(x=w1588, y=3.0) -> (x*y=w1591:dbl)
                }
                frame "s" {
                  n669 = Multiply(x=w1594, y=1000000000.0) -> (x*y=w1593:dbl)
                  n670 = Multiply(x=w1593, y=3.0) -> (x*y=w1596:dbl)
                }
              }
              n671 = Subtract(x=w1571, y=w1565) -> (x-y=w1569:dbl)
              n672 = Divide(x=w1569, y=2.0) -> (x/y=w1568:dbl)
              n673 = Multiply(x=w1572, y=w1568) -> (x*y=w1566:dbl)
              n674 = Multiply(x=w1572, y=w1570) -> (x*y=w1573:dbl)
              n675 = Less?(x=w1571, y=w1570) -> (x < y?=w1574:bool)
              n676 = Select(t=w1566, s=w1574, f=w1573) -> (s? t:f=w1562:dbl)
              n677 = Multiply(x=1e-06, y=w1562) -> (x*y=w1563:dbl)
            }
            frame "us" {
              w1609 = 0.795 ("lower limit")
              n678 = case shown="Default" w1613 {
                tunnel: w1612 -> [w1614 w1618 w1623 w1628 w1633]
                tunnel: [w1615 w1620 w1625 w1630 w1635] -> w1607
                tunnel: [w1614 w1617 w1622 w1627 w1632] -> w1602
                frame Default {
                  n679 = Multiply(x=w1614, y=3.0) -> (x*y=w1615:dbl)
                }
                frame "ns" {
                  n680 = Multiply(x=w1618, y=0.001) -> (x*y=w1617:dbl)
                  n681 = Multiply(x=w1617, y=3.0) -> (x*y=w1620:dbl)
                }
                frame "us" {
                  n682 = Multiply(x=w1623, y=1.0) -> (x*y=w1622:dbl)
                  n683 = Multiply(x=w1622, y=3.0) -> (x*y=w1625:dbl)
                }
                frame "ms" {
                  n684 = Multiply(x=w1628, y=1000.0) -> (x*y=w1627:dbl)
                  n685 = Multiply(x=w1627, y=3.0) -> (x*y=w1630:dbl)
                }
                frame "s" {
                  n686 = Multiply(x=w1633, y=1000000.0) -> (x*y=w1632:dbl)
                  n687 = Multiply(x=w1632, y=3.0) -> (x*y=w1635:dbl)
                }
              }
              n688 = Subtract(x=w1608, y=w1602) -> (x-y=w1606:dbl)
              n689 = Divide(x=w1606, y=2.0) -> (x/y=w1605:dbl)
              n690 = Multiply(x=w1609, y=w1605) -> (x*y=w1603:dbl)
              n691 = Multiply(x=w1609, y=w1607) -> (x*y=w1610:dbl)
              n692 = Less?(x=w1608, y=w1607) -> (x < y?=w1611:bool)
              n693 = Select(t=w1603, s=w1611, f=w1610) -> (s? t:f=w1600:dbl)
              n694 = Multiply(x=0.001, y=w1600) -> (x*y=w1601:dbl)
            }
            frame "ms" {
              w1648 = 0.795 ("lower limit")
              n695 = case shown="Default" w1652 {
                tunnel: w1651 -> [w1653 w1657 w1662 w1667 w1672]
                tunnel: [w1654 w1659 w1664 w1669 w1674] -> w1646
                tunnel: [w1653 w1656 w1661 w1666 w1671] -> w1641
                frame Default {
                  n696 = Multiply(x=w1653, y=3.0) -> (x*y=w1654:dbl)
                }
                frame "ns" {
                  n697 = Multiply(x=w1657, y=1e-06) -> (x*y=w1656:dbl)
                  n698 = Multiply(x=w1656, y=3.0) -> (x*y=w1659:dbl)
                }
                frame "us" {
                  n699 = Multiply(x=w1662, y=0.001) -> (x*y=w1661:dbl)
                  n700 = Multiply(x=w1661, y=3.0) -> (x*y=w1664:dbl)
                }
                frame "ms" {
                  n701 = Multiply(x=w1667, y=1.0) -> (x*y=w1666:dbl)
                  n702 = Multiply(x=w1666, y=3.0) -> (x*y=w1669:dbl)
                }
                frame "s" {
                  n703 = Multiply(x=w1672, y=1000.0) -> (x*y=w1671:dbl)
                  n704 = Multiply(x=w1671, y=3.0) -> (x*y=w1674:dbl)
                }
              }
              n705 = Subtract(x=w1647, y=w1641) -> (x-y=w1645:dbl)
              n706 = Divide(x=w1645, y=2.0) -> (x/y=w1644:dbl)
              n707 = Multiply(x=w1648, y=w1644) -> (x*y=w1642:dbl)
              n708 = Multiply(x=w1648, y=w1646) -> (x*y=w1649:dbl)
              n709 = Less?(x=w1647, y=w1646) -> (x < y?=w1650:bool)
              n710 = Select(t=w1642, s=w1650, f=w1649) -> (s? t:f=w1639:dbl)
              n711 = Multiply(x=1.0, y=w1639) -> (x*y=w1640:dbl)
            }
            frame "s" {
              w1687 = 0.795 ("lower limit")
              n712 = case shown="Default" w1691 {
                tunnel: w1690 -> [w1692 w1696 w1701 w1706 w1711]
                tunnel: [w1693 w1698 w1703 w1708 w1713] -> w1685
                tunnel: [w1692 w1695 w1700 w1705 w1710] -> w1680
                frame Default {
                  n713 = Multiply(x=w1692, y=3.0) -> (x*y=w1693:dbl)
                }
                frame "ns" {
                  n714 = Multiply(x=w1696, y=1e-06) -> (x*y=w1695:dbl)
                  n715 = Multiply(x=w1695, y=3.0) -> (x*y=w1698:dbl)
                }
                frame "us" {
                  n716 = Multiply(x=w1701, y=0.001) -> (x*y=w1700:dbl)
                  n717 = Multiply(x=w1700, y=3.0) -> (x*y=w1703:dbl)
                }
                frame "ms" {
                  n718 = Multiply(x=w1706, y=1.0) -> (x*y=w1705:dbl)
                  n719 = Multiply(x=w1705, y=3.0) -> (x*y=w1708:dbl)
                }
                frame "s" {
                  n720 = Multiply(x=w1711, y=1000.0) -> (x*y=w1710:dbl)
                  n721 = Multiply(x=w1710, y=3.0) -> (x*y=w1713:dbl)
                }
              }
              n722 = Subtract(x=w1686, y=w1680) -> (x-y=w1684:dbl)
              n723 = Divide(x=w1684, y=2.0) -> (x/y=w1683:dbl)
              n724 = Multiply(x=w1687, y=w1683) -> (x*y=w1681:dbl)
              n725 = Multiply(x=w1687, y=w1685) -> (x*y=w1688:dbl)
              n726 = Less?(x=w1686, y=w1685) -> (x < y?=w1689:bool)
              n727 = Select(t=w1681, s=w1689, f=w1688) -> (s? t:f=w1678:dbl)
              n728 = Multiply(x=1000.0, y=w1678) -> (x*y=w1679:dbl)
            }
          }
          n729 = In Range and Coerce(upper limit=w1546, x=w1553, lower limit=10.0) -> (coerced(x)=w1554:dbl, In Range?=w1547:bool)
          n730 = case shown="False" w1547 {
            tunnel: w1546 -> [w1556 _]
            tunnel: w1545 -> [w1555 _]
            frame False {
              n731 = Format Into String(format string="FallEdge time can`t be lower than 10 ns or higher than %.3f %s!" ("message"), w1556, w1555) -> (resulting string=w1558:string)  [unwired: 2 in, 1 out]
              n732 = One Button Dialog(message=w1558) -> ()  [unwired: 1 in, 1 out]
            }
            frame True {
            }
          }
        }
        frame "s" {
          n733 = case shown="\"ns\"" w1721 {
            tunnel: w1720 -> [_ w1741 w1778 w1817 w1856]
            tunnel: w1719 -> [w1730 w1745 w1782 w1821 w1860]
            tunnel: w1718 -> [_ w1746 w1783 w1822 w1861]
            tunnel: [w1730 w1733 w1771 w1810 w1849] -> w1716
            tunnel: ["ns" "ns" "us" "ms" "s"] -> w1715
            frame Default {
            }
            frame "ns" {
              w1742 = 0.795 ("lower limit")
              n734 = case shown="Default" w1746 {
                tunnel: w1745 -> [w1747 w1750 w1754 w1759 w1764]
                tunnel: [w1748 w1751 w1756 w1761 w1766] -> w1740
                tunnel: [w1747 w1750 w1753 w1758 w1763] -> w1735
                frame Default {
                  n735 = Multiply(x=w1747, y=3.0) -> (x*y=w1748:dbl)
                }
                frame "ns" {
                  n736 = Multiply(x=w1750, y=3.0) -> (x*y=w1751:dbl)
                }
                frame "us" {
                  n737 = Multiply(x=w1754, y=1000.0) -> (x*y=w1753:dbl)
                  n738 = Multiply(x=w1753, y=3.0) -> (x*y=w1756:dbl)
                }
                frame "ms" {
                  n739 = Multiply(x=w1759, y=1000000.0) -> (x*y=w1758:dbl)
                  n740 = Multiply(x=w1758, y=3.0) -> (x*y=w1761:dbl)
                }
                frame "s" {
                  n741 = Multiply(x=w1764, y=1000000000.0) -> (x*y=w1763:dbl)
                  n742 = Multiply(x=w1763, y=3.0) -> (x*y=w1766:dbl)
                }
              }
              n743 = Subtract(x=w1741, y=w1735) -> (x-y=w1739:dbl)
              n744 = Divide(x=w1739, y=2.0) -> (x/y=w1738:dbl)
              n745 = Multiply(x=w1742, y=w1738) -> (x*y=w1736:dbl)
              n746 = Multiply(x=w1742, y=w1740) -> (x*y=w1743:dbl)
              n747 = Less?(x=w1741, y=w1740) -> (x < y?=w1744:bool)
              n748 = Select(t=w1736, s=w1744, f=w1743) -> (s? t:f=w1732:dbl)
              n749 = Multiply(x=1e-09, y=w1732) -> (x*y=w1733:dbl)
            }
            frame "us" {
              w1779 = 0.795 ("lower limit")
              n750 = case shown="Default" w1783 {
                tunnel: w1782 -> [w1784 w1788 w1793 w1798 w1803]
                tunnel: [w1785 w1790 w1795 w1800 w1805] -> w1777
                tunnel: [w1784 w1787 w1792 w1797 w1802] -> w1772
                frame Default {
                  n751 = Multiply(x=w1784, y=3.0) -> (x*y=w1785:dbl)
                }
                frame "ns" {
                  n752 = Multiply(x=w1788, y=0.001) -> (x*y=w1787:dbl)
                  n753 = Multiply(x=w1787, y=3.0) -> (x*y=w1790:dbl)
                }
                frame "us" {
                  n754 = Multiply(x=w1793, y=1.0) -> (x*y=w1792:dbl)
                  n755 = Multiply(x=w1792, y=3.0) -> (x*y=w1795:dbl)
                }
                frame "ms" {
                  n756 = Multiply(x=w1798, y=1000.0) -> (x*y=w1797:dbl)
                  n757 = Multiply(x=w1797, y=3.0) -> (x*y=w1800:dbl)
                }
                frame "s" {
                  n758 = Multiply(x=w1803, y=1000000.0) -> (x*y=w1802:dbl)
                  n759 = Multiply(x=w1802, y=3.0) -> (x*y=w1805:dbl)
                }
              }
              n760 = Subtract(x=w1778, y=w1772) -> (x-y=w1776:dbl)
              n761 = Divide(x=w1776, y=2.0) -> (x/y=w1775:dbl)
              n762 = Multiply(x=w1779, y=w1775) -> (x*y=w1773:dbl)
              n763 = Multiply(x=w1779, y=w1777) -> (x*y=w1780:dbl)
              n764 = Less?(x=w1778, y=w1777) -> (x < y?=w1781:bool)
              n765 = Select(t=w1773, s=w1781, f=w1780) -> (s? t:f=w1770:dbl)
              n766 = Multiply(x=1e-06, y=w1770) -> (x*y=w1771:dbl)
            }
            frame "ms" {
              w1818 = 0.795 ("lower limit")
              n767 = case shown="Default" w1822 {
                tunnel: w1821 -> [w1823 w1827 w1832 w1837 w1842]
                tunnel: [w1824 w1829 w1834 w1839 w1844] -> w1816
                tunnel: [w1823 w1826 w1831 w1836 w1841] -> w1811
                frame Default {
                  n768 = Multiply(x=w1823, y=3.0) -> (x*y=w1824:dbl)
                }
                frame "ns" {
                  n769 = Multiply(x=w1827, y=1e-06) -> (x*y=w1826:dbl)
                  n770 = Multiply(x=w1826, y=3.0) -> (x*y=w1829:dbl)
                }
                frame "us" {
                  n771 = Multiply(x=w1832, y=0.001) -> (x*y=w1831:dbl)
                  n772 = Multiply(x=w1831, y=3.0) -> (x*y=w1834:dbl)
                }
                frame "ms" {
                  n773 = Multiply(x=w1837, y=1.0) -> (x*y=w1836:dbl)
                  n774 = Multiply(x=w1836, y=3.0) -> (x*y=w1839:dbl)
                }
                frame "s" {
                  n775 = Multiply(x=w1842, y=1000.0) -> (x*y=w1841:dbl)
                  n776 = Multiply(x=w1841, y=3.0) -> (x*y=w1844:dbl)
                }
              }
              n777 = Subtract(x=w1817, y=w1811) -> (x-y=w1815:dbl)
              n778 = Divide(x=w1815, y=2.0) -> (x/y=w1814:dbl)
              n779 = Multiply(x=w1818, y=w1814) -> (x*y=w1812:dbl)
              n780 = Multiply(x=w1818, y=w1816) -> (x*y=w1819:dbl)
              n781 = Less?(x=w1817, y=w1816) -> (x < y?=w1820:bool)
              n782 = Select(t=w1812, s=w1820, f=w1819) -> (s? t:f=w1809:dbl)
              n783 = Multiply(x=0.001, y=w1809) -> (x*y=w1810:dbl)
            }
            frame "s" {
              w1857 = 0.795 ("lower limit")
              n784 = case shown="Default" w1861 {
                tunnel: w1860 -> [w1862 w1866 w1871 w1876 w1881]
                tunnel: [w1863 w1868 w1873 w1878 w1883] -> w1855
                tunnel: [w1862 w1865 w1870 w1875 w1880] -> w1850
                frame Default {
                  n785 = Multiply(x=w1862, y=3.0) -> (x*y=w1863:dbl)
                }
                frame "ns" {
                  n786 = Multiply(x=w1866, y=1e-06) -> (x*y=w1865:dbl)
                  n787 = Multiply(x=w1865, y=3.0) -> (x*y=w1868:dbl)
                }
                frame "us" {
                  n788 = Multiply(x=w1871, y=0.001) -> (x*y=w1870:dbl)
                  n789 = Multiply(x=w1870, y=3.0) -> (x*y=w1873:dbl)
                }
                frame "ms" {
                  n790 = Multiply(x=w1876, y=1.0) -> (x*y=w1875:dbl)
                  n791 = Multiply(x=w1875, y=3.0) -> (x*y=w1878:dbl)
                }
                frame "s" {
                  n792 = Multiply(x=w1881, y=1000.0) -> (x*y=w1880:dbl)
                  n793 = Multiply(x=w1880, y=3.0) -> (x*y=w1883:dbl)
                }
              }
              n794 = Subtract(x=w1856, y=w1850) -> (x-y=w1854:dbl)
              n795 = Divide(x=w1854, y=2.0) -> (x/y=w1853:dbl)
              n796 = Multiply(x=w1857, y=w1853) -> (x*y=w1851:dbl)
              n797 = Multiply(x=w1857, y=w1855) -> (x*y=w1858:dbl)
              n798 = Less?(x=w1856, y=w1855) -> (x < y?=w1859:bool)
              n799 = Select(t=w1851, s=w1859, f=w1858) -> (s? t:f=w1848:dbl)
              n800 = Multiply(x=1.0, y=w1848) -> (x*y=w1849:dbl)
            }
          }
          n801 = In Range and Coerce(upper limit=w1716, x=w1723, lower limit=10.0) -> (coerced(x)=w1724:dbl, In Range?=w1717:bool)
          n802 = case shown="False" w1717 {
            tunnel: w1716 -> [w1726 _]
            tunnel: w1715 -> [w1725 _]
            frame False {
              n803 = Format Into String(format string="FallEdge time can`t be lower than 10 ns or higher than %.3f %s!" ("message"), w1726, w1725) -> (resulting string=w1728:string)  [unwired: 2 in, 1 out]
              n804 = One Button Dialog(message=w1728) -> ()  [unwired: 1 in, 1 out]
            }
            frame True {
            }
          }
        }
      }
      n805 = Bundle By Name(cluster=w1203, "FallEdge"=w1195) -> (w1200:T14)
      n806 = To Variant(anything=w1200) -> (Variant=w1199:variant)
    }
    frame Default {
    }
  }
  "error out" <- w4
  "Rigol DG822 Pulse out" <- w2
  "Coerced Value" <- w1
